vi "TRANCON-Client.vi"() -> ()   [LabVIEW 2020]
uses:
  controls/Rename.ctl
  controls/Load.ctl
  controls/CleanSD.ctl
  controls/Save.ctl
  controls/Del.ctl
  controls/Add.ctl
  controls/Average.ctl
  controls/mylistbox.ctl
  dependecies/XControls/StartButton/StartButton.xctl
  controls/SliderSDII.ctl
  controls/Gauge_pump/Gauge_pump.xctl
  controls/DigitalIndicatorELYSEpulses.ctl
  dependecies/XControls/CellsDL/ControlDL.xctl
  controls/Calc.ctl
  controls/Camera.ctl
  controls/table.ctl
  controls/oscilloscope.ctl
  controls/AllOffOn.ctl
  controls/Fix.ctl
  controls/Scale_up.ctl
  controls/Norm.ctl
  controls/LeftArrow.ctl
  controls/RightArrow.ctl
  controls/Visibility.ctl
  Classes/Control/Control-Client/Control-Client.lvclass
  dependecies/ControlsVIs/Clusters-def/Delays-refs_CLIENT.ctl
  dependecies/ControlsVIs/Clusters-def/graphs_TR.ctl
  dependecies/ControlsVIs/Clusters-def/Graphs_ref_Client.ctl
  dependecies/ControlsVIs/Clusters-def/Controls-with-permissions_CLIENT.ctl
  <vilib>/addons/zeromq/socket_type.ctl
  <vilib>/addons/zeromq/socket_options.ctl
  dependecies/ControlsVIs/Clusters-def/SERVER-Commands.ctl
  dependecies/ControlsVIs/Clusters-def/Message types.ctl
  Classes/Control/Control-Client/Control-Client.lvclass/Control-Client.ctl
  Classes/Experiments/Experiments_group.lvclass/Experiments_group.ctl
  dependecies/ControlsVIs/Clusters-def/Types_of_Graphs-Client.ctl
  Classes/Experiments/Experiment.lvclass/Experiment.ctl
  dependecies/ControlsVIs/Clusters-def/Parameters_measurement_def.ctl
  Classes/Control/Control-Client/methods/Read Group #.vi
  dependecies/globalVarII.vi
  dependecies/globalVarSD.vi
  Classes/Control/Control-Client/Erase color.vi
  Classes/Experiments/Experiments_group.lvclass
  Classes/Control/Control-Server/Control-Server.lvclass
  Classes/Experiments/Experiment.lvclass
  <vilib>/addons/zeromq/zmq_context.lvclass
  <vilib>/addons/zeromq/zmq_socket.lvclass
  <vilib>/addons/zeromq/zeromq.lvlib
panel:
  in  "EXP":bool=TRUE caption="EXP V0/VD2"
  in  "BG type":enum32{"Aver", "Savitzky-Golay"}(radio)=enum."Savitzky-Golay"
  out "BG":cluster{i32[], "Filtered X":dbl[]}[](graph)
  in  "polynom order":i32=10
  in  "side p":i32=10
  in  "aver":bool
  in  "Cut":bool
  in  "right exp":bool
  in  "left exp":bool=TRUE
  in  "Fix":bool
  in  "Up":bool
  in  "Left":bool
  in  "Right":bool
  in  "Numeric":i32=5 min=1 max=50
  in  "scale":dbl=1.01
  in  "timedelays_var":dbl[](array[numeric])=[370.0, 400.0, 450.0, 500.0, 550.0, 600.0, 640.0, 700.0]
  in  "waves_var":dbl[](array[numeric])=[370.0, 400.0, 450.0, 500.0, 550.0, 600.0, 640.0, 700.0]
  in  "Merge":bool
  in  "VD2_calc_abs":bool
  in  "Right shift kinetics":T1
  in  "Left shift kinetics":T2
  in  "Norm Kinetics":T3
  in  "Scale_up":dbl=1.01 format="%#_3f"
  in  "ScaleUp":T4
  in  "Value":dbl=10.0 format="%#_13g"
  in  "ChangeAll":T5
  in  "NaN Correct":T6
  in  "CalcStability":T7
  out "stability":T8(graph)
  in  "X-scale":bool
  out "bytes received":i64 caption="DATA received"
  in  "Group title":string
  in  "Del group exp":T9
  in  "Add group":T10
  out "error out":errorcluster
  in  "Exp name":string
  in  "Clean mode":u16(ring)=1 items=["delete", "approx"]
  in  "Clean":T6
  in  "sigma":dbl=1.4 min=0.0 step=0.1
  in  "BG slider":T11={0.0, 16.0} scale=0.0..15.0
  in  "BG correct":T6
  in  "Add Exp":T10
  in  "Del exp":T9
  in  "Load Exp":T12
  in  "Save exp":T13
  in  "Save":enum32{"Automatic", "User-def"}(ring)
  in  "Rename exp":T14
  in  "Average exp":T15
  in  "times slider":T11={120.7741935483871, 734.8387096774194} scale=0.0..1.0 scale format="%#.1f"
  in  "del spec":i32=2 min=2 step=1
  in  "Del spectrum":T9
  in  "Add spectrum":T10
  out "Spectra":cluster{"Y":dbl[], "Y":dbl[]}[](graph)
  in  "waves slider":T11={434.19354838709677, 734.8387096774194} scale=0.0..1.0 scale format="%#.1f"
  in  "del kin":i32=2 min=2 step=1
  in  "LogY":bool
  in  "Del kinetics":T9
  in  "Add kinetics":T10
  out "Kinetics":cluster{"Y":dbl[], "Y":dbl[]}[](graph)
  in  "Camer connect":bool
  in  "Pump connect":bool
  in  "OSc:Connect":bool
  in  "folder of the day":string="no title"
  out "Power":bool
  in  "DAQmx:Connect":bool
  in  "Unlock":bool
  in  "SERVER:AllConnect":bool caption="All connect"
  in  "DET:Connect":bool
  in  "DL:Connect":bool
  in  "StartButton":bool(xcontrol)
  in  "Server ON/OFF":bool
  in  "selected wavelengths":dbl[](array[numeric])=[370.0, 400.0, 450.0, 500.0, 550.0, 600.0, 640.0, 700.0]
  out "Exp data graph":dbl[][](graph)
  in  "Commentaires exp":string="...Write experiment description..."
  in  "Experiments":T16=[4]
  in  "Group":u16(ring)
  in  "type of probe":enum32{"SC", "OPA"}(radio)
  in  "Tab Control":enum32{"Exp data", "Raw data"}(tab)
  out "TR OD":cluster{dbl[], dbl[]}[](graph)
  in  "CalcAbs":T7
  in  "SaveSC":T13
  in  "RT":bool
  out "TR SC":cluster{dbl[], dbl[]}[](graph)
  in  "correct raw BG":bool
  out "Raw data":cluster{dbl[], dbl[]}[](graph)
  in  "raw bg":i32[](array[numeric])
  out "Raw data BG":cluster{dbl[], dbl[]}[](graph)
  out "Pump":T17(xcontrol)
  in  "visibility":T18
  in  "#cycles_measurement":i32=5 caption="#Cyc" min=1 max=15 step=1
  in  "Define Names":bool
  in  "Repump":bool
  in  "Lockrepump_levels":T19
  out "ELYSE pulses":T20
  in  "channelsOsc":i16[](array[numeric])=[1] min=0 max=3 step=1
  in  "oscilloscopeRead":T21
  out "Oscilloscope":waveform(dbl)[](graph)
  in  "image":T22
  out "Camera":dbl[][](graph)
  out "Total length, ps":dbl=3989.9999999999995 caption="Total"
  out "Kinetics length, ps":dbl=3789.9999999999995 caption="Kinetics" min=-200.0 max=8350.0
  in  "Real zero, ps":dbl=465.0 caption="Real zero"
  in  "remake":bool
  in  "# points":i32=100 min=1 step=1
  in  "OZ, ps":dbl=-250.0
  in  "Step, ps":dbl=15.0 min=-100.0 max=5000.0 step=1.0
  in  "TableLoad":T23
  out "Delays Graph":cluster{i32[], "array w/ subset deleted":dbl[]}(graph)
  in  "DAQmx:FaradayCup":bool caption="Accelerator shutter"
  out "Alarm":bool
  in  "DAQmx:RelayKeyHeater":bool caption="Accelerator shutter"
  in  "DAQmx:AcceleratorShutter":bool caption="Accelerator shutter"
  in  "DAQmx:LaserShutter":bool
  in  "Time, ms":dbl=10.0 min=1.0 max=150.0
  in  "DAQmx:MoveCrystal":bool
  in  "Start measurement":bool
  in  "Wavelength fix":dbl=640.0 caption="wave fix"
  in  "ODmax":dbl=0.5
  in  "ODmin":dbl=-0.5
  in  "# par point":i32=10 caption="# PP" min=1 max=100 step=1
  out "# current":i32 caption="#"
  out "RDT, ps":dbl=3789.9999999999995 caption="RDT"
  in  "Aq contol":enum32{"fixed", "automatic", "fixed-auto"}(radio)
  in  "ControlDL":cluster{"positions":dbl[]}(xcontrol)
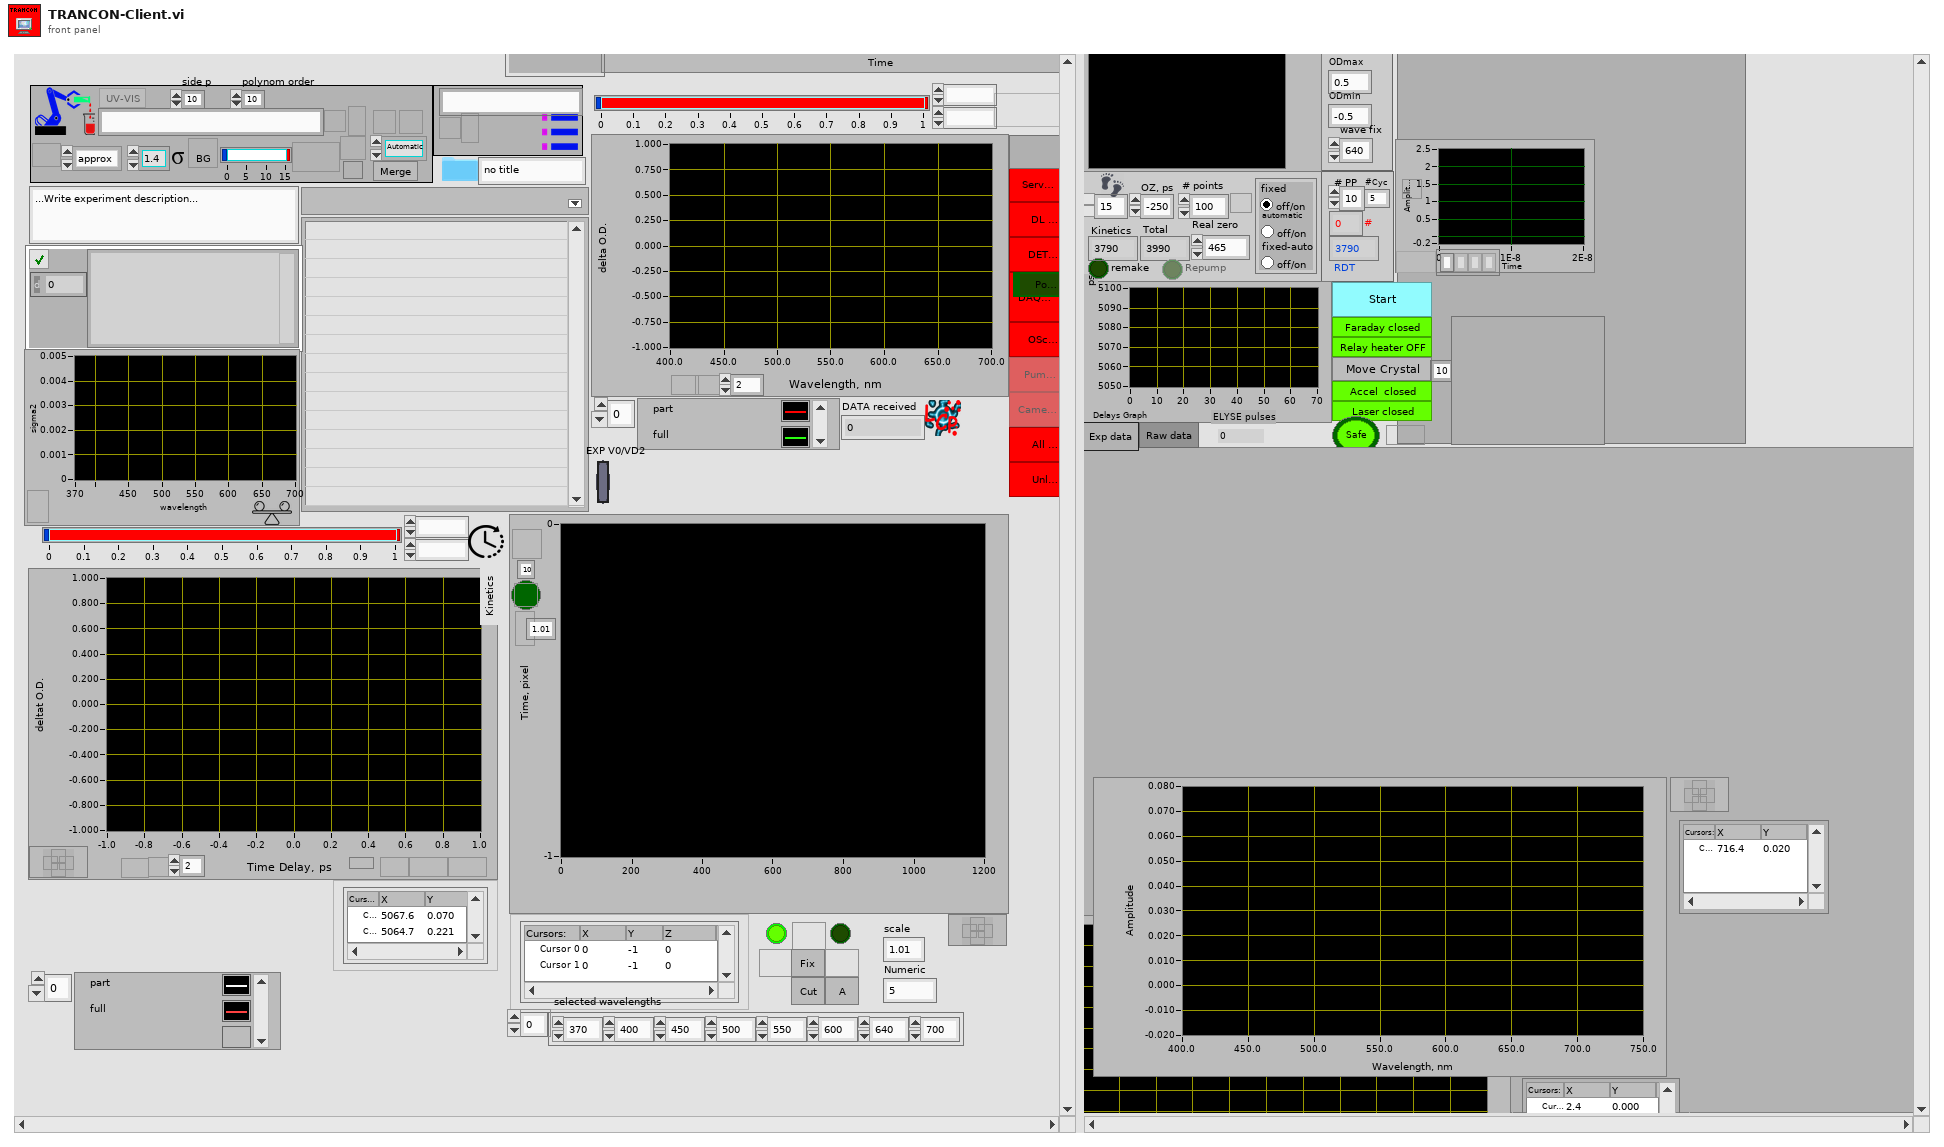
[diagram p1: front panel]
types:
  T1 = typedef "RightArrow.ctl" = bool
  T2 = typedef "LeftArrow.ctl" = bool
  T3 = typedef "Norm.ctl" = bool
  T4 = typedef "Scale_up.ctl" = bool
  T5 = typedef "AllOffOn.ctl" = bool
  T6 = typedef "CleanSD.ctl" = bool
  T7 = typedef "Calc.ctl" = bool
  T8 = cluster{"wavelengths":dbl[], "wavelengths":dbl[]}[]
  T9 = typedef "Del.ctl" = bool
  T10 = typedef "Add.ctl" = bool
  T11 = typedef "SliderSDII.ctl" = cluster{dbl, dbl}
  T12 = typedef "Load.ctl" = bool
  T13 = typedef "Save.ctl" = bool
  T14 = typedef "Rename.ctl" = bool
  T15 = typedef "Average.ctl" = bool
  T16 = typedef "mylistbox.ctl" = i32[]
  T17 = cluster{"Data":dbl, "direction":bool, "start/stop":bool}
  T18 = typedef "Visibility.ctl" = bool
  T19 = typedef "Fix.ctl" = bool
  T20 = typedef "DigitalIndicatorELYSEpulses.ctl" = i64
  T21 = typedef "oscilloscope.ctl" = bool
  T22 = typedef "Camera.ctl" = bool
  T23 = typedef "table.ctl" = bool
  T24 = cluster{"waves slider":refnum<vi>, "times slider":refnum<vi>}
  T25 = typedef "Control-Client.lvclass/Controls-with-permissions_CLIENT.ctl" = cluster{"Server ON/OFF":refnum<vi>, "Detector connect":refnum<vi>, "DL connect":refnum<vi>, "DAQmx connect":refnum<vi>, "All connect":refnum<vi>, "Start measurement":refnum<vi>, "Move Crystal":refnum<vi>, "Relay key heater":refnum<vi>, "Laser Shutter":refnum<vi>, "Accelerator Shutter":refnum<vi>, "Power":refnum<vi>, "Unlock":refnum<vi>, "RT":refnum<vi>, "Faraday Cup":refnum<vi>, "Osc connect":refnum<vi>, "ELYSE pulses":refnum<vi>, "Cells":refnum<vi>, "Pump":refnum<vi>, "# par point":refnum<vi>, "Alarm":refnum<vi>, "oscilloscopeRead":refnum<vi>, "WCM_state":refnum<vi>, "ControlDL":refnum<vi>}
  T26 = typedef "Control-Client.lvclass/Graphs_ref_Client.ctl" = cluster{"Exp data graph ref":refnum<vi>, "Kinetics graph ref":refnum<vi>, "Spectrum graph ref":refnum<vi>, "cluster graph TR":T27, "Delays Graph":refnum<vi>, "Oscilloscope":refnum<vi>}
  T27 = typedef "graphs_TR.ctl" = cluster{"TR SC":refnum<vi>, "TR OD":refnum<vi>, "Raw data":refnum<vi>, "Raw data BG":refnum<vi>}
  T28 = typedef "Control-Client.lvclass/Delays-refs_CLIENT.ctl" = cluster{"# points":refnum<vi>, "Step, ps":refnum<vi>, "OZ, ps":refnum<vi>, "# current":refnum<vi>, "RDT, ps":refnum<vi>, "Total length, ps":refnum<vi>, "Kinetics length, ps":refnum<vi>, "Real zero, ps":refnum<vi>, "# par point":refnum<vi>}
  T29 = cluster{"error out":refnum<vi>, "Experiments":refnum<vi>, "Group":refnum<vi>, "Commentaires exp":refnum<vi>}
  T30 = typedef "zeromq.lvlib/socket_options.ctl" = enum8{"NONE", "ZMQ_HWM", "<2>", "ZMQ_SWAP", "ZMQ_AFFINITY", "ZMQ_ROUTING_ID", "ZMQ_SUBSCRIBE", "ZMQ_UNSUBSCRIBE", "ZMQ_RATE", "ZMQ_RECOVERY_IVL", "ZMQ_MCAST_LOOP", "ZMQ_SNDBUF", "ZMQ_RCVBUF", "ZMQ_RCVMORE", "ZMQ_FD", "ZMQ_EVENTS", "ZMQ_TYPE", "ZMQ_LINGER", "ZMQ_RECONNECT_IVL", "ZMQ_BACKLOG", "ZMQ_RECOVERY_IVL_MSEC", "ZMQ_RECONNECT_IVL_MAX", "ZMQ_MAXMSGSIZE", "ZMQ_SNDHWM", "ZMQ_RCVHWM", "ZMQ_MULTICAST_HOPS", "<26>", "ZMQ_RCVTIMEO", "ZMQ_SNDTIMEO", "<29>", "<30>", "ZMQ_IPV4ONLY", "ZMQ_LAST_ENDPOINT", "ZMQ_ROUTER_MANDATORY", "ZMQ_TCP_KEEPALIVE", "ZMQ_TCP_KEEPALIVE_CNT", "ZMQ_TCP_KEEPALIVE_IDLE", "ZMQ_TCP_KEEPALIVE_INTVL", "ZMQ_TCP_ACCEPT_FILTER", "ZMQ_IMMEDIATE", "ZMQ_XPUB_VERBOSE", "ZMQ_ROUTER_RAW", "ZMQ_IPV6", "ZMQ_MECHANISM", "ZMQ_PLAIN_SERVER", "ZMQ_PLAIN_USERNAME", "ZMQ_PLAIN_PASSWORD", "ZMQ_CURVE_SERVER", "ZMQ_CURVE_PUBLICKEY", "ZMQ_CURVE_SECRETKEY", "ZMQ_CURVE_SERVERKEY", "ZMQ_PROBE_ROUTER", "ZMQ_REQ_CORRELATE", "ZMQ_REQ_RELAXED", "ZMQ_CONFLATE", "ZMQ_ZAP_DOMAIN", "ZMQ_ROUTER_HANDOVER", "ZMQ_TOS", "ZMQ_IPC_FILTER_PID", "ZMQ_IPC_FILTER_UID", "ZMQ_IPC_FILTER_GID", "ZMQ_CONNECT_ROUTING_ID", "ZMQ_GSSAPI_SERVER", "ZMQ_GSSAPI_PRINCIPAL", "ZMQ_GSSAPI_SERVICE_PRINCIPAL", "ZMQ_GSSAPI_PLAINTEXT", "ZMQ_HANDSHAKE_IVL", "<67>", "ZMQ_SOCKS_PROXY", "ZMQ_XPUB_NODROP", "ZMQ_BLOCKY", "ZMQ_XPUB_MANUAL", "ZMQ_XPUB_WELCOME_MSG", "ZMQ_STREAM_NOTIFY", "ZMQ_INVERT_MATCHING", "ZMQ_HEARTBEAT_IVL", "ZMQ_HEARTBEAT_TTL", "ZMQ_HEARTBEAT_TIMEOUT", "ZMQ_XPUB_VERBOSER", "ZMQ_CONNECT_TIMEOUT", "ZMQ_TCP_MAXRT", "ZMQ_THREAD_SAFE", "<82>", "<83>", "ZMQ_MULTICAST_MAXTPDU", "ZMQ_VMCI_BUFFER_SIZE", "ZMQ_VMCI_BUFFER_MIN_SIZE", "ZMQ_VMCI_BUFFER_MAX_SIZE", "ZMQ_VMCI_CONNECT_TIMEOUT", "ZMQ_USE_FD", "ZMQ_GSSAPI_PRINCIPAL_NAMETYPE", "ZMQ_GSSAPI_SERVICE_PRINCIPAL_NAMETYPE", "ZMQ_BINDTODEVICE", "ZMQ_ZAP_ENFORCE_DOMAIN", "ZMQ_LOOPBACK_FASTPATH", "ZMQ_METADATA", "ZMQ_MULTICAST_LOOP", "ZMQ_ROUTER_NOTIFY"}
  T31 = typedef "zeromq.lvlib/socket_type.ctl" = enum8{"ZMQ_PAIR", "ZMQ_PUB", "ZMQ_SUB", "ZMQ_REQ", "ZMQ_REP", "ZMQ_DEALER", "ZMQ_ROUTER", "ZMQ_PULL", "ZMQ_PUSH", "ZMQ_XPUB", "ZMQ_XSUB", "ZMQ_STREAM", "ZMQ_SERVER", "ZMQ_CLIENT", "ZMQ_RADIO", "ZMQ_DISH", "ZMQ_GATHER", "ZMQ_SCATTER", "ZMQ_DGRAM"}
  T32 = typedef "Message types.ctl" = string
  T33 = typedef "Control-Server.lvclass/SERVER-Commands.ctl" = string
  T34 = cluster{"Fix":bool, "DeltaT":dbl, "#points":i32, "Delay":dbl, "output cluster":cluster{"From Time":dbl, "To Time":dbl, "From Wave":dbl, "To Wave":dbl}}
  T35 = typedef "Control-Client.lvclass/Types_of_Graphs-Client.ctl" = string
  T36 = typedef "Parameters_measurement_def.ctl" = cluster{"ODmin":dbl, "ODmax":dbl, "Aq contol":enum32{"fixed", "automatic", "fixed-auto"}, "Wavelength_fix_index":i32, "repump_limits":cluster{"repump_min":dbl, "repump_max":dbl, "repump_value":dbl}, "repump_correction":bool, "#cycles max":i32}
  T37 = enum32{"Invalid", "Standard", "Closed", "Hidden", "Minimized", "Maximized"}
  T38 = cluster{"Value":string, "Value":string, cluster{dbl, dbl, dbl, dbl}}
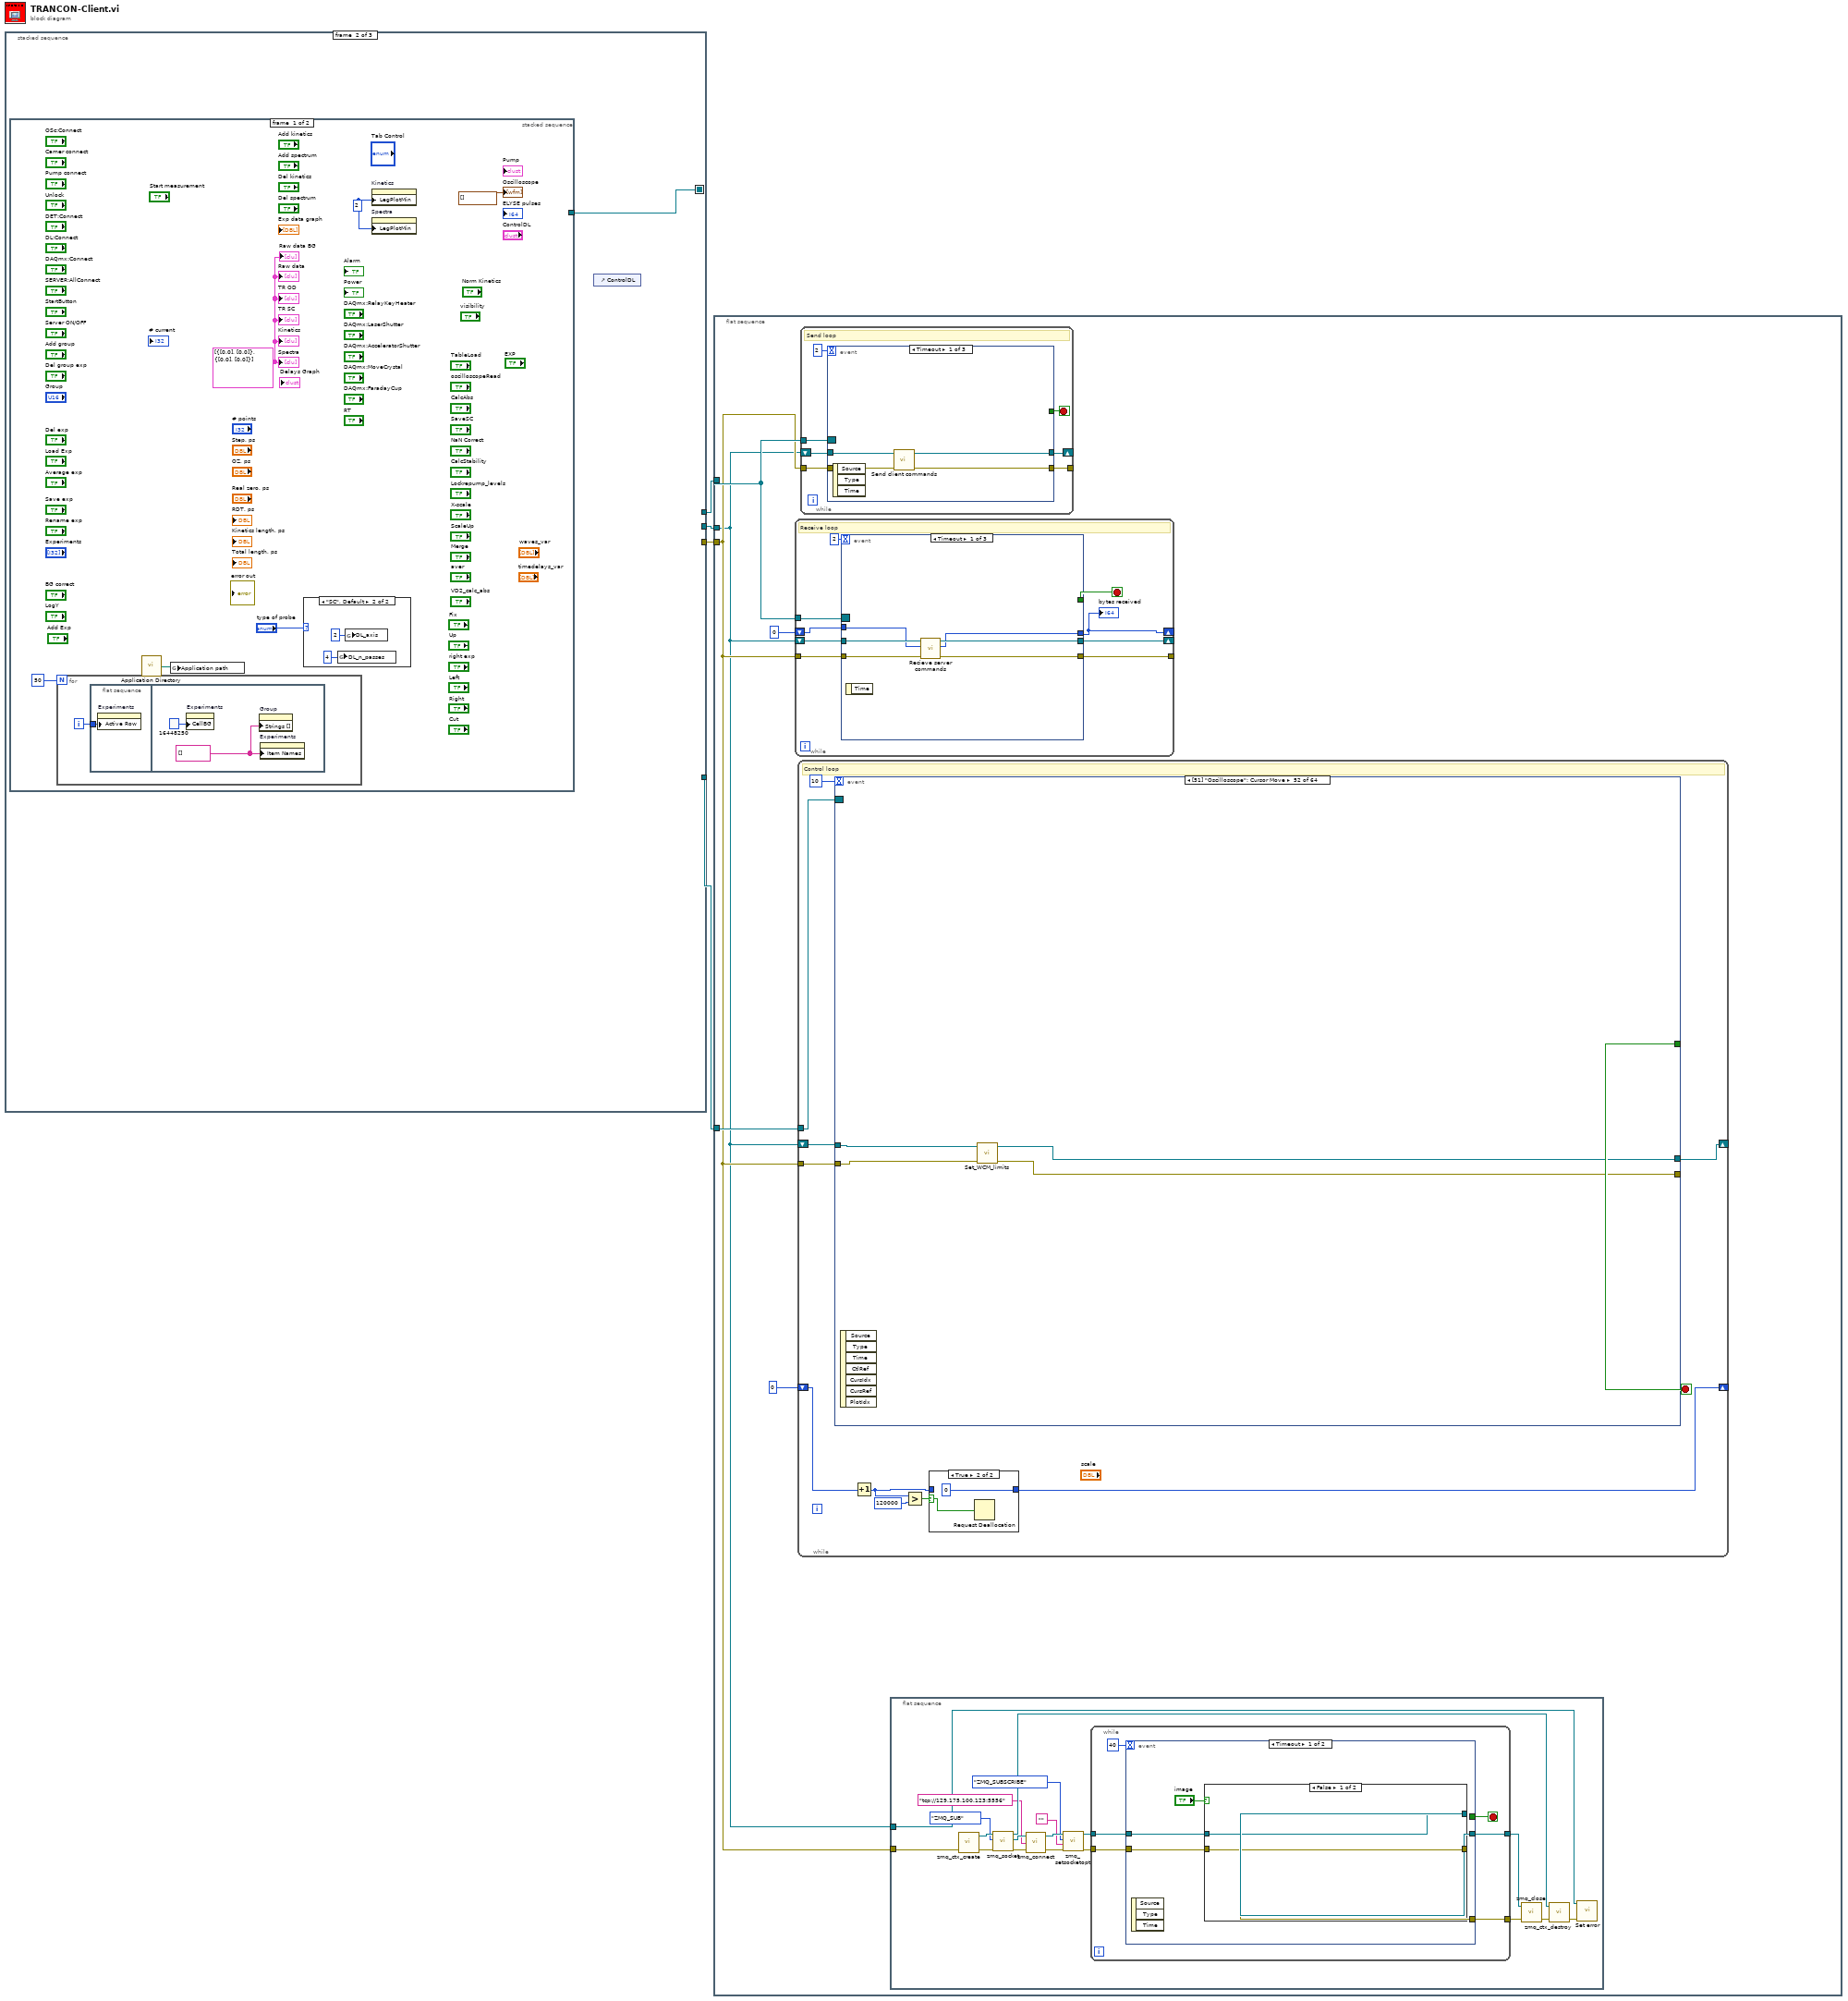
[diagram p0: block diagram]
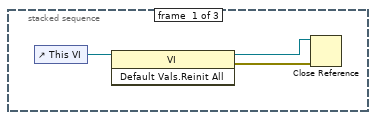
[diagram p2: hidden frame]
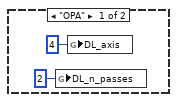
[diagram p3: hidden frame]
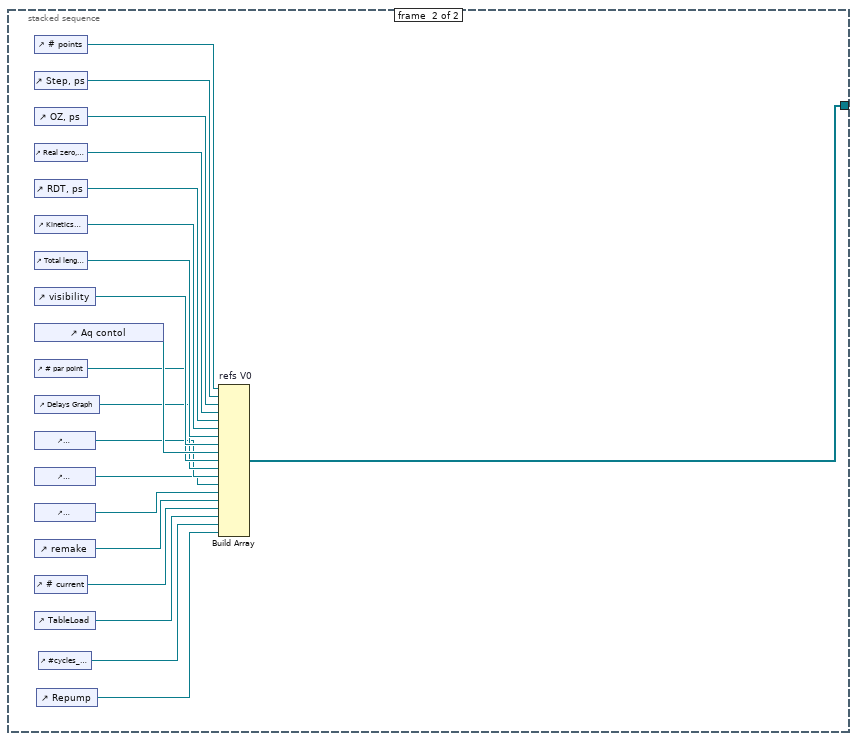
[diagram p4: hidden frame]
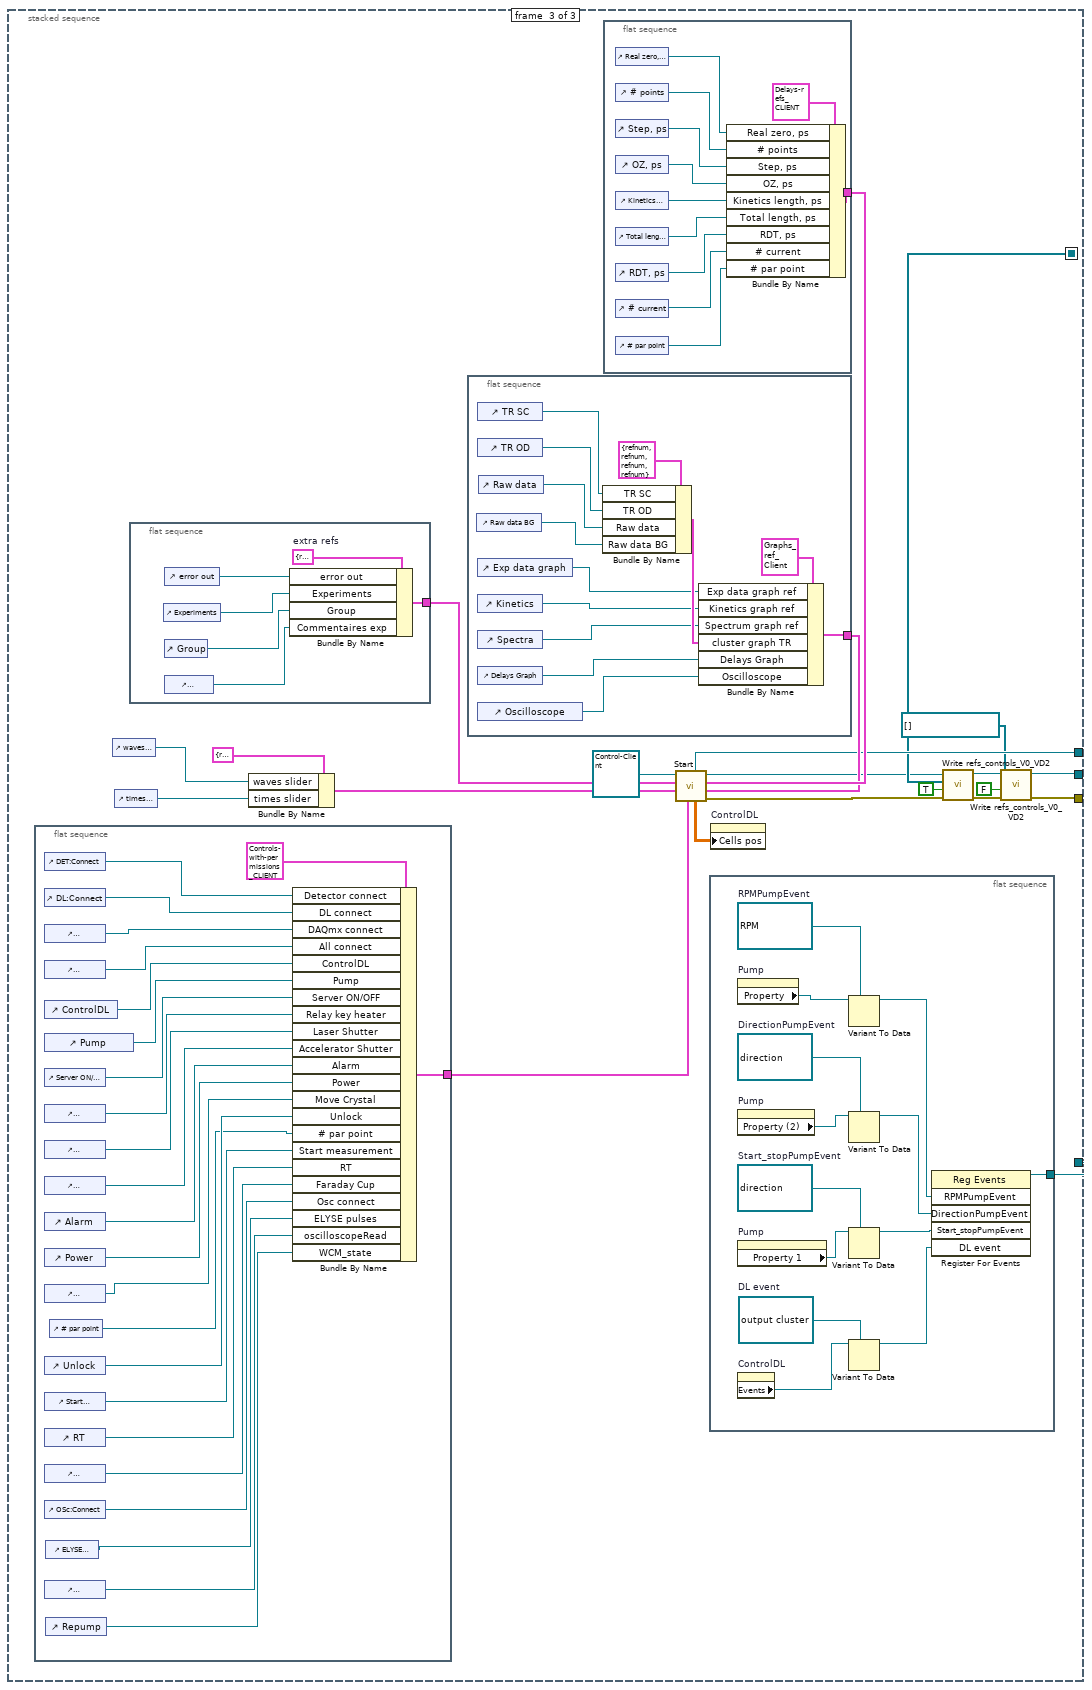
[diagram p5: hidden frame]
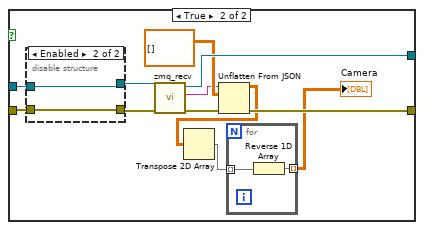
[diagram p6: hidden frame]
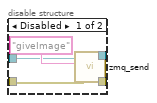
[diagram p7: hidden frame]
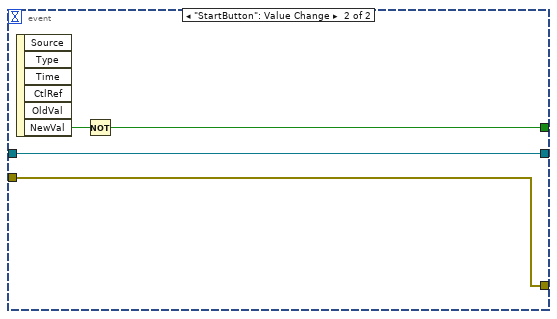
[diagram p8: hidden frame]
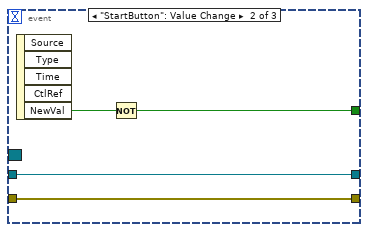
[diagram p9: hidden frame]
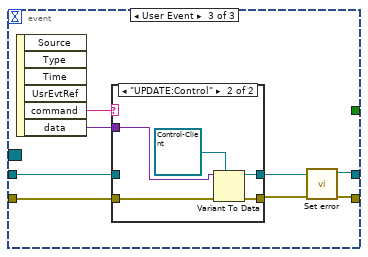
[diagram p10: hidden frame]
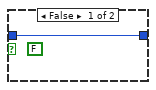
[diagram p12: hidden frame]
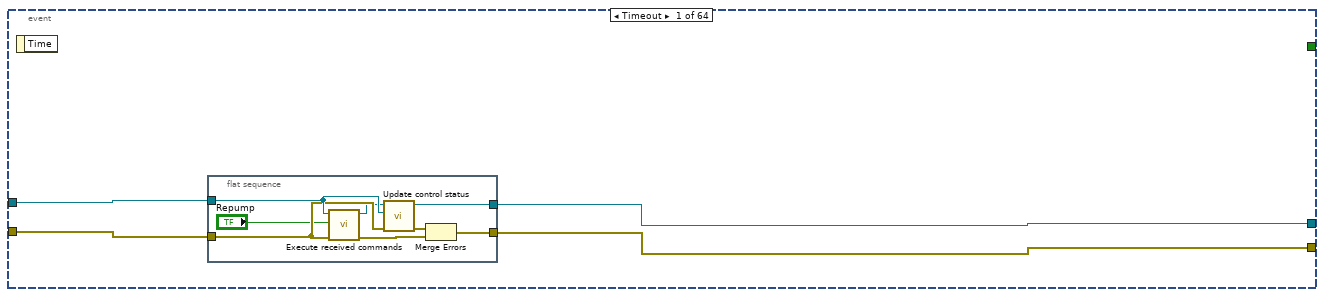
[diagram p13: hidden frame]
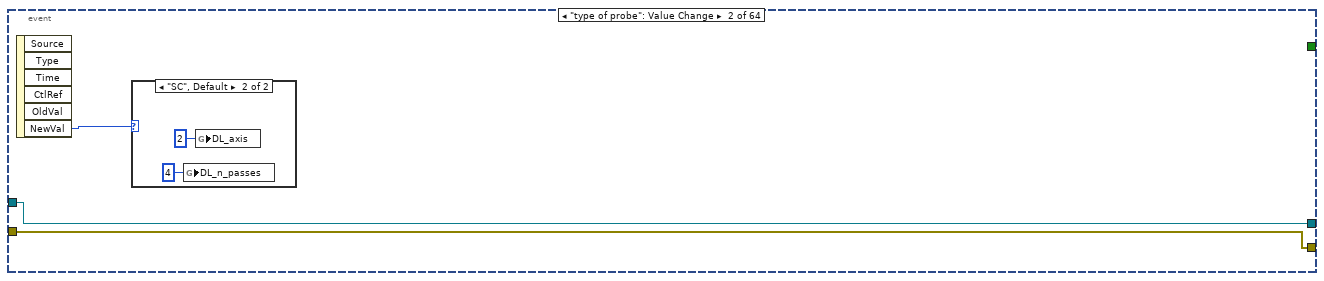
[diagram p14: hidden frame]
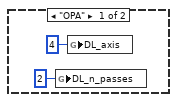
[diagram p15: hidden frame]
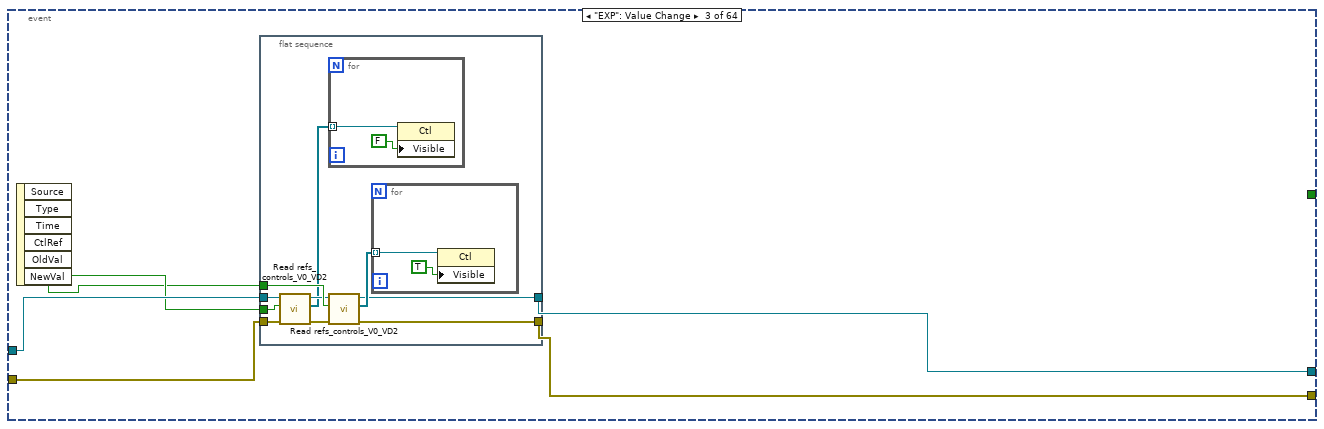
[diagram p16: hidden frame]
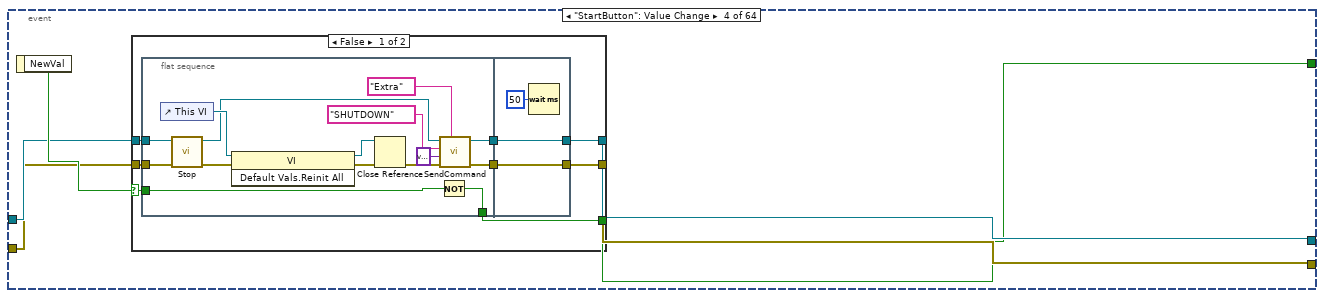
[diagram p17: hidden frame]
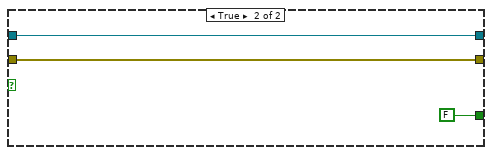
[diagram p18: hidden frame]
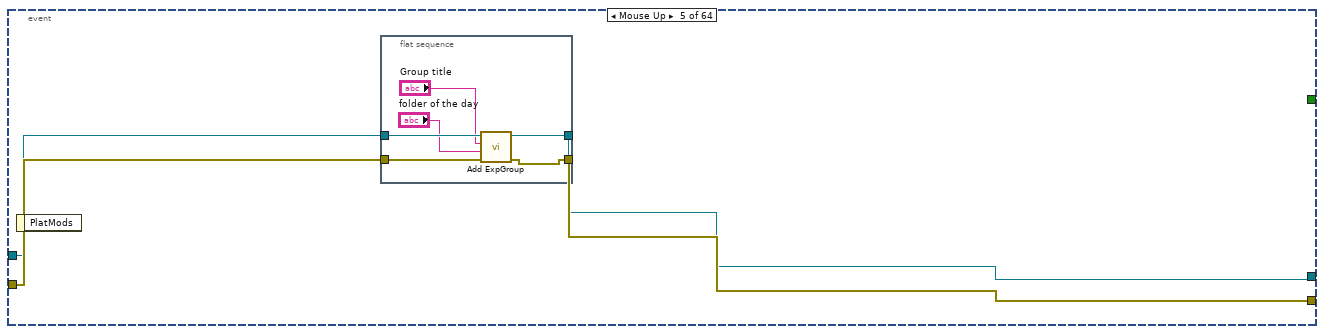
[diagram p19: hidden frame]
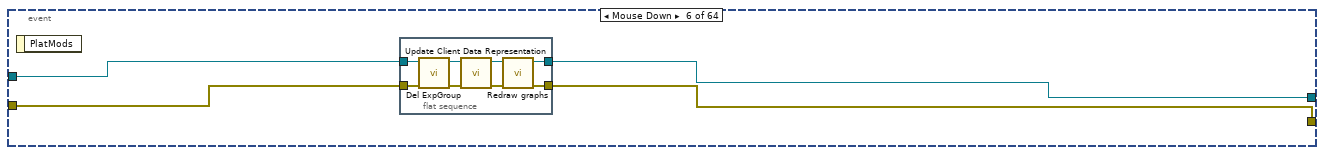
[diagram p20: hidden frame]
diagram:
  n1 = stacked-sequence {
    seq-local: [_ w8 _] -> [_ _ w51]
    tunnel: [_ _ w47] -> w4
    tunnel: [_ _ w46] -> w1
    tunnel: [_ _ w54] -> w3
    tunnel: [_ _ w62] -> w2
    frame #0 {
      n2 = control-ref of="This VI"() -> (w7:refnum<vi>)
      n3 = invoke class="VI" method="Default Vals.Reinit All"(reference=w7) -> (reference out=w6:refnum<vi>, error out=w5:errorcluster)  [unwired: 2 in, 1 out]
      n4 = Close Reference(reference=w6, error in (no error)=w5) -> ()  [unwired: 1 out]
    }
    frame #1 {
      n5 = stacked-sequence {
        tunnel: [_ w32] -> w8
        frame #0 {
          w10 = cluster{dbl[], dbl[]}[] [{[0.0], [0.0]}, {[0.0], [0.0]}] ("Kinetics")
          w12 = u32 2 ("Legend:Plot Minimum")
          n6 = for {
            N: 50 -> [_]
            i -> [w19]
            n7 = flat-sequence {
              tunnel: w19 -> [w20]
              frame #0 {
                n8 = property on="Experiments" class="LstBox (strict)"("Active Row"=w20) -> ()  [unwired: 2 in, 2 out]
              }
              frame #1 {
                w21 = string[] [] ("Item Names")
                n9 = property on="Experiments" class="LstBox (strict)"("CellBG"=u32 16448250) -> ()  [unwired: 2 in, 2 out]
                n10 = property on="Group" class="Ring (strict)"("Strings []"=w21) -> ()  [unwired: 2 in, 2 out]
                n11 = property on="Experiments" class="LstBox (strict)"("Item Names"=w21) -> ()  [unwired: 2 in, 2 out]
              }
            }
          }
          n12 = call <vilib>:"Application Directory.vi"() -> ("Application Directory"=w14:path)
          n13 = global write "globalVarSD.vi" "Application path"(w14) -> ()
          n14 = case shown="\"SC\", Default" "type of probe" {
            frame "OPA" {
              n15 = global write "globalVarII.vi" "DL_n_passes"(2 ("DL_n_passes")) -> ()
              n16 = global write "globalVarII.vi" "DL_axis"(4 ("DL_axis")) -> ()
            }
            frame "SC", Default {
              n17 = global write "globalVarII.vi" "DL_n_passes"(4 ("DL_n_passes")) -> ()
              n18 = global write "globalVarII.vi" "DL_axis"(2 ("DL_axis")) -> ()
            }
          }
          n19 = property on="Kinetics" class="XYGraph (strict)"("LegPlotMin"=w12) -> ()  [unwired: 2 in, 2 out]
          n20 = property on="Spectra" class="XYGraph (strict)"("LegPlotMin"=w12) -> ()  [unwired: 2 in, 2 out]
          "TR OD" <- w10
          "TR SC" <- w10
          "Spectra" <- w10
          "Kinetics" <- w10
          "Oscilloscope" <- waveform(dbl)[] [] ("Data")
          "Raw data" <- w10
          "Raw data BG" <- w10
        }
        frame #1 {
          n21 = control-ref of="# points"() -> (w42:refnum<vi>)
          n22 = control-ref of="Step, ps"() -> (w41:refnum<vi>)
          n23 = control-ref of="OZ, ps"() -> (w40:refnum<vi>)
          n24 = control-ref of="Real zero, ps"() -> (w39:refnum<vi>)
          n25 = control-ref of="RDT, ps"() -> (w38:refnum<vi>)
          n26 = control-ref of="Kinetics length, ps"() -> (w37:refnum<vi>)
          n27 = control-ref of="Total length, ps"() -> (w36:refnum<vi>)
          n28 = control-ref of="visibility"() -> (w35:refnum<vi>)
          n29 = control-ref of="Aq contol"() -> (w34:refnum<vi>)
          n30 = control-ref of="# par point"() -> (w33:refnum<vi>)
          n31 = control-ref of="Delays Graph"() -> (w31:refnum<vi>)
          n32 = control-ref of="DAQmx:MoveCrystal"() -> (w30:refnum<vi>)
          n33 = control-ref of="DAQmx:AcceleratorShutter"() -> (w29:refnum<vi>)
          n34 = control-ref of="DAQmx:LaserShutter"() -> (w28:refnum<vi>)
          n35 = control-ref of="remake"() -> (w27:refnum<vi>)
          n36 = control-ref of="# current"() -> (w26:refnum<vi>)
          n37 = control-ref of="TableLoad"() -> (w25:refnum<vi>)
          n38 = control-ref of="Repump"() -> (w23:refnum<vi>)
          n39 = control-ref of="#cycles_measurement"() -> (w24:refnum<vi>)
          n40 = Build Array "refs V0"(w42, w41, w40, w39, w38, w37, w36, w35, w34, w33, w31, w30, w29, w28, w27, w26, w25, w24, w23) -> (w32:refnum<vi>[])
        }
      }
      n41 = control-ref of="ControlDL"() -> ()  [unwired: 1 out]
    }
    frame #2 {
      n42 = flat-sequence {
        tunnel: [w71] -> w57
        frame #0 {
          n43 = control-ref of="DET:Connect"() -> (w94:refnum<vi>)
          n44 = control-ref of="DL:Connect"() -> (w93:refnum<vi>)
          n45 = control-ref of="DAQmx:Connect"() -> (w92:refnum<vi>)
          n46 = control-ref of="SERVER:AllConnect"() -> (w91:refnum<vi>)
          n47 = control-ref of="ControlDL"() -> (w78:refnum<vi>)
          n48 = control-ref of="Pump"() -> (w77:refnum<vi>)
          n49 = control-ref of="Server ON/OFF"() -> (w90:refnum<vi>)
          n50 = control-ref of="DAQmx:RelayKeyHeater"() -> (w89:refnum<vi>)
          n51 = control-ref of="DAQmx:LaserShutter"() -> (w88:refnum<vi>)
          n52 = control-ref of="DAQmx:AcceleratorShutter"() -> (w87:refnum<vi>)
          n53 = control-ref of="Alarm"() -> (w75:refnum<vi>)
          n54 = control-ref of="Power"() -> (w86:refnum<vi>)
          n55 = control-ref of="DAQmx:MoveCrystal"() -> (w85:refnum<vi>)
          n56 = control-ref of="Unlock"() -> (w83:refnum<vi>)
          n57 = control-ref of="Start measurement"() -> (w82:refnum<vi>)
          n58 = control-ref of="RT"() -> (w81:refnum<vi>)
          n59 = control-ref of="DAQmx:FaradayCup"() -> (w80:refnum<vi>)
          n60 = control-ref of="OSc:Connect"() -> (w79:refnum<vi>)
          n61 = control-ref of="oscilloscopeRead"() -> (w74:refnum<vi>)
          n62 = control-ref of="ELYSE pulses"() -> (w73:refnum<vi>)
          n63 = control-ref of="Repump"() -> (w72:refnum<vi>)
          n64 = control-ref of="# par point"() -> (w76:refnum<vi>)
          n65 = Bundle By Name(cluster=T25 {"Server ON/OFF"=refnum, "Detector connect"=refnum, "DL connect"=refnum, "DAQmx connect"=refnum, "All connect"=refnum, "Start measurement"=refnum, "Move Crystal"=refnum, "Relay key heater"=refnum, "Laser Shutter"=refnum, "Accelerator Shutter"=refnum, "Power"=refnum, "Unlock"=refnum, "RT"=refnum, "Faraday Cup"=refnum, "Osc connect"=refnum, "ELYSE pulses"=refnum, "Cells"=refnum, "Pump"=refnum, "# par point"=refnum, "Alarm"=refnum, "oscilloscopeRead"=refnum, "WCM_state"=refnum, "ControlDL"=refnum} ("output cluster"), "Detector connect"=w94, "DL connect"=w93, "DAQmx connect"=w92, "All connect"=w91, "ControlDL"=w78, "Pump"=w77, "Server ON/OFF"=w90, "Relay key heater"=w89, "Laser Shutter"=w88, "Accelerator Shutter"=w87, "Alarm"=w75, "Power"=w86, "Move Crystal"=w85, "Unlock"=w83, "# par point"=w76, "Start measurement"=w82, "RT"=w81, "Faraday Cup"=w80, "Osc connect"=w79, "ELYSE pulses"=w73, "oscilloscopeRead"=w74, "WCM_state"=w72) -> (w71:T25)
        }
      }
      n66 = control-ref of="waves slider"() -> (w60:refnum<vi>)
      n67 = control-ref of="times slider"() -> (w61:refnum<vi>)
      n68 = flat-sequence {
        tunnel: [w65] -> w55
        frame #0 {
          w70 = T29 {"error out"=refnum, "Experiments"=refnum, "Group"=refnum, "Commentaires exp"=refnum}  # extra refs
          n69 = control-ref of="Experiments"() -> (w68:refnum<vi>)
          n70 = control-ref of="error out"() -> (w69:refnum<vi>)
          n71 = control-ref of="Group"() -> (w67:refnum<vi>)
          n72 = control-ref of="Commentaires exp"() -> (w66:refnum<vi>)
          n73 = Bundle By Name(cluster=w70, "error out"=w69, "Experiments"=w68, "Group"=w67, "Commentaires exp"=w66) -> (w65:T29)
        }
      }
      n74 = Bundle By Name(cluster=T24 {"waves slider"=refnum, "times slider"=refnum}, "waves slider"=w60, "times slider"=w61) -> (w59:T24)
      n75 = flat-sequence {
        tunnel: [w103] -> w56
        frame #0 {
          n76 = control-ref of="Raw data BG"() -> (w95:refnum<vi>)
          n77 = control-ref of="TR SC"() -> (w106:refnum<vi>)
          n78 = control-ref of="TR OD"() -> (w105:refnum<vi>)
          n79 = control-ref of="Exp data graph"() -> (w98:refnum<vi>)
          n80 = control-ref of="Kinetics"() -> (w100:refnum<vi>)
          n81 = control-ref of="Spectra"() -> (w99:refnum<vi>)
          n82 = control-ref of="Delays Graph"() -> (w101:refnum<vi>)
          n83 = control-ref of="Oscilloscope"() -> (w97:refnum<vi>)
          n84 = control-ref of="Raw data"() -> (w96:refnum<vi>)
          n85 = Bundle By Name(cluster=T27 {"TR SC"=refnum, "TR OD"=refnum, "Raw data"=refnum, "Raw data BG"=refnum} ("cluster de sortie"), "TR SC"=w106, "TR OD"=w105, "Raw data"=w96, "Raw data BG"=w95) -> (w102:T27)
          n86 = Bundle By Name(cluster=T26 {"Exp data graph ref"=refnum, "Kinetics graph ref"=refnum, "Spectrum graph ref"=refnum, "cluster graph TR"={"TR SC"=refnum, "TR OD"=refnum, "Raw data"=refnum, "Raw data BG"=refnum}, "Delays Graph"=refnum, "Oscilloscope"=refnum} ("Graph refs"), "Exp data graph ref"=w98, "Kinetics graph ref"=w100, "Spectrum graph ref"=w99, "cluster graph TR"=w102, "Delays Graph"=w101, "Oscilloscope"=w97) -> (w103:T26)
        }
      }
      n87 = flat-sequence {
        tunnel: [w109] -> w58
        frame #0 {
          n88 = control-ref of="Real zero, ps"() -> (w113:refnum<vi>)
          n89 = control-ref of="# points"() -> (w114:refnum<vi>)
          n90 = control-ref of="Step, ps"() -> (w115:refnum<vi>)
          n91 = control-ref of="OZ, ps"() -> (w116:refnum<vi>)
          n92 = control-ref of="Kinetics length, ps"() -> (w117:refnum<vi>)
          n93 = control-ref of="Total length, ps"() -> (w118:refnum<vi>)
          n94 = control-ref of="RDT, ps"() -> (w111:refnum<vi>)
          n95 = control-ref of="# current"() -> (w110:refnum<vi>)
          n96 = control-ref of="# par point"() -> (w108:refnum<vi>)
          n97 = Bundle By Name(cluster=T28 {"# points"=refnum, "Step, ps"=refnum, "OZ, ps"=refnum, "# current"=refnum, "RDT, ps"=refnum, "Total length, ps"=refnum, "Kinetics length, ps"=refnum, "Real zero, ps"=refnum, "# par point"=refnum}, "Real zero, ps"=w113, "# points"=w114, "Step, ps"=w115, "OZ, ps"=w116, "Kinetics length, ps"=w117, "Total length, ps"=w118, "RDT, ps"=w111, "# current"=w110, "# par point"=w108) -> (w109:T28)
        }
      }
      n98 = call "Start.vi"("Graph refs"=w56, "Delays refs"=w58, "buttons refs"=w57, "Slider cluster"=w59, "extra refs"=w55, "Control-Client in"=refnum<class "Control-Client.lvclass"> refnum) -> ("error out"=w52:errorcluster, "Control-Client out"=w49:refnum<class "Control-Client.lvclass">, "preset pos"=w53:dbl[][], "ControlEventCom event"=w54:refnum<event-registration>)  [unwired: 2 in]
      n99 = flat-sequence {
        tunnel: [w131] -> w62
        frame #0 {
          w119 = refnum<user-event> refnum  # DL event
          w124 = refnum<user-event> refnum  # Start_stopPumpEvent
          w127 = refnum<user-event> refnum  # DirectionPumpEvent
          w129 = refnum<user-event> refnum  # RPMPumpEvent
          n100 = property on="Pump" class="Gauge_pump (strict)"() -> ("Property"=w130:refnum<user-event>)  [unwired: 2 in, 2 out]
          n101 = property on="Pump" class="Gauge_pump (strict)"() -> ("Property (2)"=w126:refnum<user-event>)  [unwired: 2 in, 2 out]
          n102 = property on="Pump" class="Gauge_pump (strict)"() -> ("Property 1"=w123:refnum<user-event>)  [unwired: 2 in, 2 out]
          n103 = property on="ControlDL" class="ControlDL (strict)"() -> ("Events"=w120:refnum<user-event>)  [unwired: 2 in, 2 out]
          n104 = Variant To Data(type=w129, Variant=w130) -> (data=w128:refnum<user-event>)  [unwired: 1 in, 1 out]
          n105 = Variant To Data(type=w127, Variant=w126) -> (data=w125:refnum<user-event>)  [unwired: 1 in, 1 out]
          n106 = Variant To Data(type=w124, Variant=w123) -> (data=w122:refnum<user-event>)  [unwired: 1 in, 1 out]
          n107 = Variant To Data(type=w119, Variant=w120) -> (data=w121:refnum<user-event>)  [unwired: 1 in, 1 out]
          n108 = register-events(w128, w125, w122, w121) -> (reference out=w131:refnum<event-registration>)  [unwired: 2 in, 1 out]
        }
      }
      n109 = property on="ControlDL" class="ControlDL (strict)"("Cells pos"=w53) -> ()  [unwired: 2 in, 2 out]
      n110 = call-dynamic "Write refs_controls_V0_VD2.vi"("error in (no error)"=w52, "EXP"=TRUE, "refs_controls_V0"=w51, "Control-Client in"=w49) -> ("error out"=w48:errorcluster, "Control-Client out"=w45:refnum<class "Control-Client.lvclass">)  [unwired: 6 in]
      n111 = call-dynamic "Write refs_controls_V0_VD2.vi"("error in (no error)"=w48, "EXP"=FALSE, "refs_controls_V0"=refnum<vi>[] [], "Control-Client in"=w45) -> ("error out"=w47:errorcluster, "Control-Client out"=w46:refnum<class "Control-Client.lvclass">)  [unwired: 6 in]
    }
  }
  n112 = flat-sequence {
    tunnel: w4 -> [w135]
    tunnel: w1 -> [w134]
    tunnel: w3 -> [w137]
    tunnel: w2 -> [w136]
    frame #0 {
      n113 = while {
        shift-right: [w1162] -> _
        shift-left: w134 -> [w1165]
        tunnel: w137 -> [w1161]
        tunnel: w135 -> [w1164]
        tunnel: [w1163] -> _
        shift-right: [w1158] -> _
        shift-left: 0 -> [w1159]
        stop <- w1166 stop-if-true
        # "Receive loop"
        n114 = event shown="[0] Timeout" {
          selector: w1161 -> [_ _ _]
          dyn-events: _ -> [_ _ _]
          timeout: 2 -> [_ _ _]
          tunnel: [_ w1174 _] -> w1166
          tunnel: w1165 -> [w1172 w1177 w1184]
          tunnel: w1164 -> [w1171 w1176 w1183]
          tunnel: [w1169 w1176 w1179] -> w1163
          tunnel: [w1170 w1177 w1180] -> w1162
          tunnel: [w1167 w1173 w1178] -> w1158
          tunnel: w1159 -> [w1168 w1173 w1178]
          event Timeout {
            n115 = event-data() -> ()  [unwired: 1 in, 1 out]
            n116 = call "Recieve server commands.vi"("error in (no error)"=w1171, "bytes in"=w1168, "Control-Client in"=w1172) -> ("error out"=w1169:errorcluster, "bytes out"=w1167:i64, "Control-Client out"=w1170:refnum<class "Control-Client.lvclass">)  [unwired: 6 in]
          }
          event "StartButton": Value Change {
            n117 = event-data() -> ("NewVal"=w1175:bool)  [unwired: 1 in, 4 out]
            n118 = Not(x=w1175) -> (.not. x?=w1174:bool)
          }
          event User Event {
            n119 = event-data() -> ("command"=w1185:string, "data"=w1186:variant)  [unwired: 1 in, 4 out]
            n120 = case shown="\"UPDATE:Control\"" w1185 {
              tunnel: w1186 -> [_ w1192]
              tunnel: [w1188 w1191] -> w1182
              tunnel: w1184 -> [w1188 _]
              tunnel: w1183 -> [w1187 w1190]
              tunnel: [w1187 w1189] -> w1181
              frame "False", Default {
              }
              frame "UPDATE:Control" {
                n121 = Variant To Data(error in=w1190, type=refnum<class "Control-Client.lvclass"> refnum ("Control-Client.lvclass"), Variant=w1192) -> (data=w1191:refnum<class "Control-Client.lvclass">, error out=w1189:errorcluster)
              }
            }
            n122 = call "Set error.vi"("error in (no error)"=w1181, "Control-Client in"=w1182) -> ("error out"=w1179:errorcluster, "Control-Client out"=w1180:refnum<class "Control-Client.lvclass">)  [unwired: 8 in]
          }
        }
        "bytes received" <- w1158
      }
      n123 = while "Control Loop" {
        tunnel: w135 -> [w235]
        shift-right: [w230] -> _
        shift-left: w134 -> [w234]
        tunnel: w136 -> [w231]
        shift-right: [w226] -> _
        shift-left: 0 -> [w228]
        stop <- w233 stop-if-true
        # "Control loop"
        n124 = event shown="[51] \"Oscilloscope\": Cursor Move" {
          selector: w231 -> [_ _ _ _ _ _ _ _ _ _ _ _ _ _ _ _ _ _ _ _ _ _ _ _ _ _ _ _ _ _ _ _ _ _ _ _ _ _ _ _ _ _ _ _ _ _ _ _ _ _ _ _ _ _ _ _ _ _ _ _ _ _ _ _]
          dyn-events: _ -> [_ _ _ _ _ _ _ _ _ _ _ _ _ _ _ _ _ _ _ _ _ _ _ _ _ _ _ _ _ _ _ _ _ _ _ _ _ _ _ _ _ _ _ _ _ _ _ _ _ _ _ _ _ _ _ _ _ _ _ _ _ _ _ _]
          timeout: 10 -> [_ _ _ _ _ _ _ _ _ _ _ _ _ _ _ _ _ _ _ _ _ _ _ _ _ _ _ _ _ _ _ _ _ _ _ _ _ _ _ _ _ _ _ _ _ _ _ _ _ _ _ _ _ _ _ _ _ _ _ _ _ _ _ _]
          tunnel: w235 -> [w240 w251 w263 w279 w316 w326 w338 w365 w378 w387 w402 w415 w427 w444 w450 w469 w474 w479 w489 w501 w511 w528 w561 w574 w586 w596 w599 w605 w615 w639 w677 w689 w718 w734 w749 w762 w780 w799 w807 w819 w825 w845 w868 w883 w905 w922 w926 w930 w957 w971 w983 w992 w995 w1002 w1035 w1039 w1054 w1064 w1086 w1095 w1120 w1135 w1139 w1149]
          tunnel: [w241 w251 w258 w280 w315 w324 w336 w367 w376 w388 w400 w416 w430 w443 w447 w468 w471 w478 w488 w500 w512 w524 w559 w572 w585 w596 w599 w604 w614 w637 w678 w690 w719 w733 w747 w760 w778 w799 w806 w817 w824 w844 w866 w881 w904 w922 w925 w929 w955 w968 w980 w990 w996 w1001 w1034 w1038 w1055 w1066 w1086 w1096 w1119 w1132 w1138 w1148] -> _
          tunnel: w234 -> [w242 w252 w262 w281 w314 w325 w339 w364 w379 w390 w403 w418 w428 w445 w449 w470 w475 w480 w490 w502 w514 w526 w562 w575 w587 w597 w600 w606 w616 w640 w680 w692 w721 w735 w750 w763 w781 w800 w804 w820 w826 w846 w869 w884 w906 w923 w927 w931 w958 w970 w984 w993 w998 w1003 w1036 w1041 w1052 w1065 w1087 w1098 w1121 w1134 w1136 w1151]
          tunnel: [w239 w252 w259 w282 w313 w323 w337 w366 w377 w389 w401 w417 w429 w442 w448 w467 w473 w476 w487 w499 w513 w525 w560 w573 w588 w597 w600 w603 w613 w638 w679 w691 w720 w732 w748 w761 w779 w800 w805 w818 w823 w843 w867 w880 w903 w923 w924 w928 w956 w969 w981 w991 w997 w1004 w1033 w1040 w1053 w1067 w1087 w1097 w1118 w1133 w1137 w1147] -> w230
          tunnel: [_ _ _ w278 _ _ _ _ _ _ _ _ _ _ _ _ _ _ _ _ _ _ _ _ _ _ _ _ _ _ _ _ _ _ _ _ _ _ _ _ _ _ _ _ _ _ _ _ _ _ _ _ _ _ _ _ _ _ _ _ _ _ _ _] -> w233
          event Timeout {
            n125 = event-data() -> ()  [unwired: 1 in, 1 out]
            n126 = flat-sequence {
              tunnel: [w250] -> w239
              tunnel: w242 -> [w249]
              tunnel: [w248] -> w241
              tunnel: w240 -> [w247]
              frame #0 {
                n127 = call "Execute received commands.vi"("error in (no error)"=w247, "repump"="Repump", "Control-Client in"=w249) -> ("error out"=w244:errorcluster, "Control-Client out"=w246:refnum<class "Control-Client.lvclass">)  [unwired: 7 in]
                n128 = call "Update control status.vi"("error in (no error)"=w247, "Control-Client old"=w249, "Control-Client new"=w246) -> ("error out"=w245:errorcluster, "Control-Client en sortie"=w250:refnum<class "Control-Client.lvclass">)  [unwired: 7 in]
                n129 = Merge Errors(w245, w244) -> (w248:errorcluster)
              }
            }
          }
          event "type of probe": Value Change {
            n130 = event-data() -> ("NewVal"=w253:enum32{"SC", "OPA"})  [unwired: 1 in, 5 out]
            n131 = case shown="\"SC\", Default" w253 {
              frame "OPA" {
                n132 = global write "globalVarII.vi" "DL_n_passes"(2 ("DL_n_passes")) -> ()
                n133 = global write "globalVarII.vi" "DL_axis"(4 ("DL_axis")) -> ()
              }
              frame "SC", Default {
                n134 = global write "globalVarII.vi" "DL_n_passes"(4 ("DL_n_passes")) -> ()
                n135 = global write "globalVarII.vi" "DL_axis"(2 ("DL_axis")) -> ()
              }
            }
          }
          event "EXP": Value Change {
            n136 = event-data() -> ("OldVal"=w261:bool, "NewVal"=w260:bool)  [unwired: 1 in, 4 out]
            n137 = flat-sequence {
              tunnel: w263 -> [w273]
              tunnel: w262 -> [w272]
              tunnel: w261 -> [w271]
              tunnel: w260 -> [w270]
              tunnel: [w265] -> w259
              tunnel: [w264] -> w258
              frame #0 {
                n138 = call-dynamic "Read refs_controls_V0_VD2.vi"("error in (no error)"=w273, "EXP"=w271, "Control-Client in"=w272) -> ("error out"=w268:errorcluster, "refs_controls"=w267:refnum<vi>[], "Control-Client out"=w269:refnum<class "Control-Client.lvclass">)  [unwired: 6 in]
                n139 = for {
                  tunnel: w267 -> [w277] mode=indexing
                  n140 = property class="Ctl"(reference=w277, "Visible"=FALSE) -> ()  [unwired: 1 in, 2 out]
                }
                n141 = call-dynamic "Read refs_controls_V0_VD2.vi"("error in (no error)"=w268, "EXP"=w270, "Control-Client in"=w269) -> ("error out"=w264:errorcluster, "refs_controls"=w266:refnum<vi>[], "Control-Client out"=w265:refnum<class "Control-Client.lvclass">)  [unwired: 6 in]
                n142 = for {
                  tunnel: w266 -> [w275] mode=indexing
                  n143 = property class="Ctl"(reference=w275, "Visible"=TRUE) -> ()  [unwired: 1 in, 2 out]
                }
              }
            }
          }
          event "StartButton": Value Change {
            n144 = event-data() -> ("NewVal"=w283:bool)  [unwired: 1 in]
            n145 = case shown="False" w283 {
              selector: w283 -> [w289 _]
              tunnel: [w287 w310] -> w282
              tunnel: w281 -> [w291 w310]
              tunnel: [w285 w311] -> w280
              tunnel: w279 -> [w290 w311]
              tunnel: [w288 FALSE] -> w278
              frame False {
                n146 = flat-sequence {
                  tunnel: w291 -> [w306]
                  tunnel: w290 -> [w305]
                  tunnel: w289 -> [w304]
                  tunnel: [w295] -> w288
                  tunnel: [w294] -> w286
                  tunnel: [w293] -> w284
                  tunnel: [w309] -> w287
                  tunnel: w286 -> [w309]
                  tunnel: [w308] -> w285
                  tunnel: w284 -> [w308]
                  frame #0 {
                    n147 = control-ref of="This VI"() -> (w301:refnum<vi>)
                    n148 = call-dynamic "Stop.vi"("error in (no error)"=w305, "Control-Client in"=w306) -> ("error out"=w300:errorcluster, "Control-Client out"=w296:refnum<class "Control-Client.lvclass">)  [unwired: 8 in]
                    n149 = invoke class="VI" method="Default Vals.Reinit All"(reference=w301, error in=w300) -> (reference out=w302:refnum<vi>, error out=w303:errorcluster)  [unwired: 1 in, 1 out]
                    n150 = Close Reference(reference=w302, error in (no error)=w303) -> (error out=w297:errorcluster)
                    n151 = Not(x=w304) -> (.not. x?=w295:bool)
                    n152 = call "SendCommand.vi"("Message type"=T32 "Extra", "error in (no error)"=w297, "data"=variant, "Command"=T33 "SHUTDOWN" ("Commands"), "Control-Client in"=w296) -> ("error out"=w293:errorcluster, "Control-Client out"=w294:refnum<class "Control-Client.lvclass">)  [unwired: 5 in]
                  }
                  frame #1 {
                    n153 = Wait (ms)(milliseconds to wait=u32 50) -> ()  [unwired: 1 out]
                  }
                }
              }
              frame True {
              }
            }
          }
          event Mouse Up {
            n154 = event-data() -> ()  [unwired: 1 in, 1 out]
            n155 = flat-sequence {
              tunnel: w316 -> [w322]
              tunnel: [w318] -> w315
              tunnel: w314 -> [w321]
              tunnel: [w319] -> w313
              frame #0 {
                n156 = call "Add ExpGroup.vi"("error in (no error)"=w322, "folder of the day"="folder of the day", "Group title"="Group title", "Control-Client in"=w321) -> ("error out"=w318:errorcluster, "Control-Client out"=w319:refnum<class "Control-Client.lvclass">)  [unwired: 6 in]
              }
            }
          }
          event Mouse Down {
            n157 = event-data() -> ()  [unwired: 1 in, 1 out]
            n158 = flat-sequence {
              tunnel: w326 -> [w334]
              tunnel: w325 -> [w333]
              tunnel: [w332] -> w324
              tunnel: [w331] -> w323
              frame #0 {
                n159 = call "Del ExpGroup.vi"("error in (no error)"=w334, "Control-Client in"=w333) -> ("error out"=w327:errorcluster, "Control-Client out"=w328:refnum<class "Control-Client.lvclass">)  [unwired: 8 in]
                n160 = call "Update Client Data Representation.vi"("error in (no error)"=w327, "Control-Client in"=w328) -> ("error out"=w330:errorcluster, "Control-Client out"=w329:refnum<class "Control-Client.lvclass">)  [unwired: 8 in]
                n161 = call "Redraw graphs.vi"("error in (no error)"=w330, "Control-Client in"=w329) -> ("error out"=w332:errorcluster, "Control-Client out"=w331:refnum<class "Control-Client.lvclass">)  [unwired: 8 in]
              }
            }
          }
          event Value Change {
            n162 = event-data() -> ("NewVal"=w335:T10)  [unwired: 1 in]
            n163 = case shown="True" w335 {
              tunnel: w339 -> [w341 w363]
              tunnel: w338 -> [w340 w362]
              tunnel: [w341 w361] -> w337
              tunnel: [w340 w360] -> w336
              frame False {
              }
              frame True {
                n164 = local read "waves slider"() -> (w349:T11)
                n165 = local read "times slider"() -> (w346:T11)
                n166 = Unbundle(w346) -> (w345:dbl, w344:dbl)
                n167 = Unbundle(w349) -> (w348:dbl, w347:dbl)
                n168 = local read "# points"() -> (w359:i32)
                n169 = local read "Step, ps"() -> (w358:dbl)
                n170 = local read "OZ, ps"() -> (w357:dbl)
                n171 = Bundle "bounds"(w345, w344, w348, w347) -> (w353:cluster{dbl, dbl, dbl, dbl})  [unwired: 1 in]
                n172 = Bundle By Name(cluster=T34 {"Fix"=TRUE, "DeltaT"=0.0, "#points"=0, "Delay"=0.0, "output cluster"={"From Time"=0.0, "To Time"=0.0, "From Wave"=0.0, "To Wave"=0.0}}, "DeltaT"=w358, "#points"=w359, "Delay"=w357, "output cluster"=w353) -> (w342:T34)
                n173 = call "Add Exp.vi"("Parameters"=w342, "error in (no error)"=w362, "Exp name"="Exp name", "Commentaires exp"="Commentaires exp", "Control-Client in"=w363) -> ("error out"=w354:errorcluster, "Control-Client out"=w355:refnum<class "Control-Client.lvclass">)  [unwired: 5 in]
                n174 = call "Update Client Data Representation.vi"("error in (no error)"=w354, "Control-Client in"=w355) -> ("error out"=w352:errorcluster, "Control-Client out"=w351:refnum<class "Control-Client.lvclass">)  [unwired: 8 in]
                n175 = call "Redraw graphs.vi"("error in (no error)"=w352, "Control-Client in"=w351) -> ("error out"=w360:errorcluster, "Control-Client out"=w361:refnum<class "Control-Client.lvclass">)  [unwired: 8 in]
              }
            }
          }
          event Mouse Up {
            n176 = event-data() -> ()  [unwired: 1 in, 1 out]
            n177 = flat-sequence {
              tunnel: [w375] -> w367
              tunnel: [w374] -> w366
              tunnel: w365 -> [w373]
              tunnel: w364 -> [w372]
              frame #0 {
                n178 = call "Del Exp.vi"("error in (no error)"=w373, "Control-Client in"=w372) -> ("error out"=w370:errorcluster, "Control-Client out"=w371:refnum<class "Control-Client.lvclass">)  [unwired: 8 in]
                n179 = call "Update Client Data Representation.vi"("error in (no error)"=w370, "Control-Client in"=w371) -> ("error out"=w369:errorcluster, "Control-Client out"=w368:refnum<class "Control-Client.lvclass">)  [unwired: 8 in]
                n180 = call "Redraw graphs.vi"("error in (no error)"=w369, "Control-Client in"=w368) -> ("error out"=w375:errorcluster, "Control-Client out"=w374:refnum<class "Control-Client.lvclass">)  [unwired: 8 in]
              }
            }
          }
          event Mouse Up {
            n181 = event-data() -> ()  [unwired: 1 in, 1 out]
            n182 = flat-sequence {
              tunnel: w379 -> [w386]
              tunnel: w378 -> [w385]
              tunnel: [w384] -> w377
              tunnel: [w383] -> w376
              frame #0 {
                n183 = local read "Exp name"() -> (w382:string)
                n184 = call "Rename Exp.vi"("error in (no error)"=w385, "New exp name"=w382, "Control-Client in"=w386) -> ("error out"=w380:errorcluster, "Control-Client out"=w381:refnum<class "Control-Client.lvclass">)  [unwired: 7 in]
                n185 = call "Update Client Data Representation.vi"("error in (no error)"=w380, "Control-Client in"=w381) -> ("error out"=w383:errorcluster, "Control-Client out"=w384:refnum<class "Control-Client.lvclass">)  [unwired: 8 in]
              }
            }
          }
          event Value Change {
            n186 = event-data() -> ("NewVal"=w391:T13)  [unwired: 1 in]
            n187 = case shown="True" w391 {
              tunnel: w390 -> [w393 w398]
              tunnel: [w393 w397] -> w389
              tunnel: [w392 w394] -> w388
              tunnel: w387 -> [w392 w396]
              frame False {
              }
              frame True {
                n188 = call "Save exp.vi"("error in (no error)"=w396, "save"="Save", "Control-Client in"=w398) -> ("error out"=w394:errorcluster, "Control-Client out"=w397:refnum<class "Control-Client.lvclass">)  [unwired: 7 in]
              }
            }
          }
          event Value Change {
            n189 = event-data() -> ("NewVal"=w399:T12)  [unwired: 1 in]
            n190 = case shown="True" w399 {
              tunnel: w403 -> [w405 w414]
              tunnel: w402 -> [w404 w413]
              tunnel: [w405 w407] -> w401
              tunnel: [w404 w408] -> w400
              frame False {
              }
              frame True {
                n191 = call "Load exp.vi"("error in (no error)"=w413, "Files of Type"=string[][] [["*.dat", "DAT"], ["*.zip", "ZIP RAW"], ["*.img", "IMG"], ["*.his", "HIS"], ["*.*", "All Files"]], "Control-Client in"=w414) -> ("error out"=w410:errorcluster, "Control-Client out"=w411:refnum<class "Control-Client.lvclass">)  [unwired: 7 in]
                n192 = call "Update Client Data Representation.vi"("error in (no error)"=w410, "Control-Client in"=w411) -> ("error out"=w409:errorcluster, "Control-Client out"=w412:refnum<class "Control-Client.lvclass">)  [unwired: 8 in]
                n193 = call "Redraw graphs.vi"("error in (no error)"=w409, "Control-Client in"=w412) -> ("error out"=w408:errorcluster, "Control-Client out"=w407:refnum<class "Control-Client.lvclass">)  [unwired: 8 in]
              }
            }
          }
          event Value Change {
            n194 = event-data() -> ("NewVal"=w419:T7)  [unwired: 1 in]
            n195 = case shown="True" w419 {
              tunnel: [w421 w424] -> w417
              tunnel: w418 -> [w421 w423]
              tunnel: [w420 w425] -> w416
              tunnel: w415 -> [w420 w426]
              frame False {
              }
              frame True {
                n196 = call "CalcStability.vi"("error in (no error)"=w426, "Control-Client in"=w423) -> ("error out"=w425:errorcluster, "stability"=→"stability":T8, "Control-Client out"=w424:refnum<class "Control-Client.lvclass">)  [unwired: 7 in]
              }
            }
          }
          event "Group": Value Change {
            n197 = event-data() -> ("NewVal"=w431:u16)  [unwired: 1 in]
            n198 = flat-sequence {
              tunnel: w431 -> [w436]
              tunnel: [w432] -> w430
              tunnel: [w433] -> w429
              tunnel: w428 -> [w438]
              tunnel: w427 -> [w437]
              frame #0 {
                n199 = call "Write Group #.vi"("error in (no error)"=w437, "Group #"=w436, "Control-Client in"=w438) -> ("error out"=w440:errorcluster, "Control-Client out"=w439:refnum<class "Control-Client.lvclass">)  [unwired: 7 in]
                n200 = call "Update Client Data Representation.vi"("error in (no error)"=w440, "Control-Client in"=w439) -> ("error out"=w435:errorcluster, "Control-Client out"=w434:refnum<class "Control-Client.lvclass">)  [unwired: 8 in]
                n201 = call "Redraw graphs.vi"("error in (no error)"=w435, "Control-Client in"=w434) -> ("error out"=w432:errorcluster, "Control-Client out"=w433:refnum<class "Control-Client.lvclass">)  [unwired: 8 in]
              }
            }
          }
          event Edit Cell {
            n202 = event-data() -> ("Row"=w441:i32, "String"=w446:string)  [unwired: 1 in]
            n203 = call "Update name of exp.vi"("error in (no error)"=w444, "Exp name"=w446, "Exp #"=w441, "Control-Client in"=w445) -> ("error out"=w443:errorcluster, "Control-Client out"=w442:refnum<class "Control-Client.lvclass">)  [unwired: 6 in]
          }
          event Double Click {
            n204 = event-data() -> ("Row"=w451:i32)  [unwired: 1 in]
            n205 = stacked-sequence {
              tunnel: w451 -> [w464]
              tunnel: w450 -> [w462]
              tunnel: w449 -> [w461]
              tunnel: [w452] -> w448
              tunnel: [w453] -> w447
              frame #0 {
                n206 = call "Read Element of Exp Groups.vi"("error in (no error)"=w462, "Control-Client in"=w461) -> ("error out"=w463:errorcluster, "Experiments_group.lvclass"=w465:refnum<class "Experiments_group.lvclass">, "Control-Client out"=w459:refnum<class "Control-Client.lvclass">)  [unwired: 7 in]
                n207 = call "Set Exp sel #.vi"("error in (no error)"=w463, "Exp sel #"=w464, "Experiments_group in"=w465) -> ("error out"=w458:errorcluster, "Experiments_group out"=w460:refnum<class "Experiments_group.lvclass">)  [unwired: 7 in]
                n208 = call "Write Element of Exp Groups.vi"("error in (no error)"=w458, "Experiments_group.lvclass"=w460, "Control-Client in"=w459) -> ("error out"=w457:errorcluster, "Control-Client out"=w456:refnum<class "Control-Client.lvclass">)  [unwired: 7 in]
                n209 = call "Update Client Data Representation.vi"("error in (no error)"=w457, "Control-Client in"=w456) -> ("error out"=w454:errorcluster, "Control-Client out"=w455:refnum<class "Control-Client.lvclass">)  [unwired: 8 in]
                n210 = call "Redraw graphs.vi"("error in (no error)"=w454, "Control-Client in"=w455) -> ("error out"=w453:errorcluster, "Control-Client out"=w452:refnum<class "Control-Client.lvclass">)  [unwired: 8 in]
              }
            }
          }
          event "Commentaires exp": Value Change {
            n211 = event-data() -> ("NewVal"=w466:string)  [unwired: 1 in]
            n212 = call "Update comments exp.vi"("error in (no error)"=w469, "Commentaires"=w466, "Control-Client in"=w470) -> ("error out"=w468:errorcluster, "Control-Client out"=w467:refnum<class "Control-Client.lvclass">)  [unwired: 7 in]
          }
          event "Exp data graph": Cursor Move {
            n213 = event-data() -> ()  [unwired: 1 in, 1 out]
            n214 = call "Redraw graphs.vi"("error in (no error)"=w474, "ChangeAll"="ChangeAll", "Control-Client in"=w475) -> ("error out"=w471:errorcluster, "Control-Client out"=w473:refnum<class "Control-Client.lvclass">)  [unwired: 7 in]
          }
          event "Exp data graph": Shortcut Menu Selection (User) {
            n215 = event-data() -> ("ItemTag"=w477:string)  [unwired: 1 in]
            n216 = flat-sequence {
              tunnel: w480 -> [w486]
              tunnel: w479 -> [w485]
              tunnel: [w484] -> w478
              tunnel: [w483] -> w476
              tunnel: w477 -> [w482]
              frame #0 {
                n217 = call "Copy exp data.vi"("error in (no error)"=w485, "selected wavelengths"="selected wavelengths", "ItemTag"=w482, "Control-Client in"=w486) -> ("error out"=w484:errorcluster, "Control-Client out"=w483:refnum<class "Control-Client.lvclass">)  [unwired: 6 in]
              }
            }
          }
          event Value Change {
            n218 = event-data() -> ("NewVal"=w491:T10)  [unwired: 1 in]
            n219 = case shown="True" w491 {
              tunnel: w490 -> [w493 w498]
              tunnel: w489 -> [w492 w497]
              tunnel: [w492 w496] -> w488
              tunnel: [w493 w495] -> w487
              frame False {
              }
              frame True {
                n220 = call "Add graph.vi"("error in (no error)"=w497, "Combo Box"="Kinetics", "Control-Client in"=w498) -> ("error out"=w496:errorcluster, "Control-Client out"=w495:refnum<class "Control-Client.lvclass">)  [unwired: 7 in]
              }
            }
          }
          event Value Change {
            n221 = event-data() -> ("NewVal"=w503:T10)  [unwired: 1 in]
            n222 = case shown="True" w503 {
              tunnel: w502 -> [w505 w510]
              tunnel: w501 -> [w504 w509]
              tunnel: [w504 w508] -> w500
              tunnel: [w505 w507] -> w499
              frame False {
              }
              frame True {
                n223 = call "Add graph.vi"("error in (no error)"=w509, "Combo Box"="Spectra", "Control-Client in"=w510) -> ("error out"=w508:errorcluster, "Control-Client out"=w507:refnum<class "Control-Client.lvclass">)  [unwired: 7 in]
              }
            }
          }
          event Value Change {
            n224 = event-data() -> ("NewVal"=w515:T3)  [unwired: 1 in, 5 out]
            n225 = case shown="True" w515 {
              tunnel: w514 -> [w517 w523]
              tunnel: [w517 w522] -> w513
              tunnel: [w516 w521] -> w512
              tunnel: w511 -> [w516 w520]
              frame False {
              }
              frame True {
                n226 = local read "del kin"() -> (w518:i32)
                n227 = call "Norm graph.vi"("error in (no error)"=w520, "#kinetics"=w518, "Combo Box"="Kinetics", "Control-Client in"=w523) -> ("error out"=w521:errorcluster, "Control-Client out"=w522:refnum<class "Control-Client.lvclass">)  [unwired: 6 in]
              }
            }
          }
          event Value Change {
            n228 = event-data() -> ("CtlRef"=w529:refnum<vi>, "NewVal"=w527:variant)  [unwired: 1 in]
            n229 = flat-sequence {
              tunnel: w529 -> [w539]
              tunnel: w528 -> [w538]
              tunnel: w527 -> [w537]
              tunnel: w526 -> [w534]
              tunnel: [w533] -> w525
              tunnel: [w532] -> w524
              frame #0 {
                n230 = property class="Bool (strict)"(reference=w539, error in=w538) -> (error out=w536:errorcluster, "ClassName"=w530:string)  [unwired: 1 out]
                n231 = case shown="\"Boolean\"" w530 {
                  tunnel: [TRUE w554] -> w535
                  tunnel: [w552 w557] -> w531
                  tunnel: w537 -> [_ w556]
                  tunnel: w536 -> [w552 w555]
                  frame "Digital", Default {
                    (unwired) FALSE
                  }
                  frame "Boolean" {
                    n232 = Variant To Data(error in=w555, type=TRUE, Variant=w556) -> (data=w554:bool, error out=w557:errorcluster)
                  }
                }
                n233 = case shown="True" w535 {
                  tunnel: w534 -> [w541 w549]
                  tunnel: [w541 w548] -> w533
                  tunnel: [w540 w547] -> w532
                  tunnel: w531 -> [w540 w546]
                  frame False {
                  }
                  frame True {
                    n234 = local read "del kin"() -> (w545:i32)
                    n235 = case shown="False" "Left shift kinetics" {
                      tunnel: [0.5 -0.5] -> w542
                      frame False {
                      }
                      frame True {
                      }
                    }
                    n236 = call "Shift X kinetics.vi"("shift"=w542, "error in (no error)"=w546, "#kinetics"=w545, "Combo Box"="Kinetics", "Control-Client in"=w549) -> ("error out"=w547:errorcluster, "Control-Client out"=w548:refnum<class "Control-Client.lvclass">)  [unwired: 5 in]
                  }
                }
              }
            }
          }
          event Value Change {
            n237 = event-data() -> ("NewVal"=w563:T9)  [unwired: 1 in]
            n238 = case shown="True" w563 {
              tunnel: w562 -> [w565 w571]
              tunnel: w561 -> [w564 w570]
              tunnel: [w565 w568] -> w560
              tunnel: [w564 w567] -> w559
              frame False {
              }
              frame True {
                n239 = call "Del graph.vi"("error in (no error)"=w570, "selected graph"="del kin", "Combo Box"="Kinetics", "Control-Client in"=w571) -> ("error out"=w567:errorcluster, "Control-Client out"=w568:refnum<class "Control-Client.lvclass">)  [unwired: 6 in]
              }
            }
          }
          event Value Change {
            n240 = event-data() -> ("NewVal"=w576:T9)  [unwired: 1 in]
            n241 = case shown="True" w576 {
              tunnel: w575 -> [w578 w584]
              tunnel: w574 -> [w577 w583]
              tunnel: [w578 w581] -> w573
              tunnel: [w577 w580] -> w572
              frame False {
              }
              frame True {
                n242 = call "Del graph.vi"("error in (no error)"=w583, "selected graph"="del spec", "Combo Box"="Spectra", "Control-Client in"=w584) -> ("error out"=w580:errorcluster, "Control-Client out"=w581:refnum<class "Control-Client.lvclass">)  [unwired: 6 in]
              }
            }
          }
          event "Kinetics": Shortcut Menu Selection (User) {
            n243 = event-data() -> ("ItemTag"=w589:string)  [unwired: 1 in]
            n244 = flat-sequence {
              tunnel: w589 -> [w595]
              tunnel: [w593] -> w588
              tunnel: w587 -> [w592]
              tunnel: w586 -> [w591]
              tunnel: [w590] -> w585
              frame #0 {
                n245 = call "Copy from XY graph.vi"("error in (no error)"=w591, "ItemTag"=w595, "Type of graph"="Kinetics" ("Combo Box"), "Control-Client in"=w592) -> ("error out"=w590:errorcluster, "Control-Client out"=w593:refnum<class "Control-Client.lvclass">)  [unwired: 6 in]
              }
            }
          }
          event "Spectra": Plot Attribute Change {
            n246 = event-data() -> ("PlotIdx"=w598:i32)  [unwired: 1 in]
            n247 = property on="Spectra" class="XYGraph (strict)"("Active Plot"=w598) -> ()  [unwired: 2 in, 2 out]
          }
          event "Kinetics": Plot Attribute Change {
            n248 = event-data() -> ("PlotIdx"=w601:i32)  [unwired: 1 in]
            n249 = property on="Kinetics" class="XYGraph (strict)"("Active Plot"=w601) -> ()  [unwired: 2 in, 2 out]
          }
          event "Spectra": Shortcut Menu Selection (User) {
            n250 = event-data() -> ("ItemTag"=w602:string)  [unwired: 1 in]
            n251 = flat-sequence {
              tunnel: w606 -> [w612]
              tunnel: w605 -> [w611]
              tunnel: [w610] -> w604
              tunnel: [w609] -> w603
              tunnel: w602 -> [w608]
              frame #0 {
                n252 = call "Copy from XY graph.vi"("error in (no error)"=w611, "ItemTag"=w608, "Type of graph"=T35 "Spectra" ("Combo Box"), "Control-Client in"=w612) -> ("error out"=w610:errorcluster, "Control-Client out"=w609:refnum<class "Control-Client.lvclass">)  [unwired: 6 in]
              }
            }
          }
          event Value Change {
            n253 = event-data() -> ("NewVal"=w617:T15)  [unwired: 1 in]
            n254 = case shown="True" w617 {
              tunnel: [w619 w633] -> w613
              tunnel: w616 -> [w619 w634]
              tunnel: w615 -> [w618 w631]
              tunnel: [w618 w632] -> w614
              frame False {
              }
              frame True {
                n255 = local read "waves slider"() -> (w627:T11)
                n256 = local read "times slider"() -> (w624:T11)
                n257 = property on="Commentaires exp" class="Str"() -> ("Value"=w630:string)  [unwired: 2 in, 2 out]
                n258 = property on="Exp name" class="Str"() -> ("Value"=w629:string)  [unwired: 2 in, 2 out]
                n259 = Unbundle(w624) -> (w623:dbl, w622:dbl)
                n260 = Unbundle(w627) -> (w626:dbl, w625:dbl)
                n261 = Bundle "bounds"(w623, w622, w626, w625) -> (w621:cluster{dbl, dbl, dbl, dbl})  [unwired: 1 in]
                n262 = Bundle("Value"=w629, "Value"=w630, w621) -> (w620:T38)  [unwired: 1 in]
                n263 = call "Average experiments.vi"("error in (no error)"=w631, "sigma"="sigma", "Name+Comments+bounds"=w620, "Control-Client in"=w634) -> ("error out"=w632:errorcluster, "Control-Client out"=w633:refnum<class "Control-Client.lvclass">)  [unwired: 6 in]
              }
            }
          }
          event "side p", "polynom order": Value Change {
            n264 = event-data() -> ("CtlRef"=w636:refnum<vi>, "NewVal"=w635:variant)  [unwired: 1 in]
            n265 = flat-sequence {
              tunnel: w640 -> [w652]
              tunnel: w639 -> [w646]
              tunnel: [w644] -> w638
              tunnel: [w648] -> w637
              tunnel: w636 -> [w651]
              tunnel: w635 -> [w641]
              frame #0 {
                n266 = flat-sequence {
                  tunnel: [w653] -> w642
                  tunnel: w641 -> [w653]
                  frame #0 {
                    n267 = global write "globalVarSD.vi" "BG type"("BG type") -> ()
                    n268 = global write "globalVarSD.vi" "side points BG"("side p") -> ()
                    n269 = global write "globalVarSD.vi" "polynom order BG"("polynom order") -> ()
                  }
                }
                n270 = property class="Ctl"(reference=w651) -> ("ClassName"=w650:string)  [unwired: 1 in, 2 out]
                n271 = case shown="\"Boolean\"" w650 {
                  tunnel: [FALSE w675] -> w649
                  tunnel: w642 -> [_ w676]
                  tunnel: [TRUE w674] -> w647
                  tunnel: w646 -> [w669 w673]
                  tunnel: [w669 w672] -> w645
                  frame "Digital", Default {
                  }
                  frame "Boolean" {
                    w675 = TRUE
                    n272 = Variant To Data(error in=w673, type=w675, Variant=w676) -> (data=w674:bool, error out=w672:errorcluster)
                  }
                }
                n273 = case shown="True" w647 {
                  tunnel: w652 -> [w660 w668]
                  tunnel: w645 -> [w659 w667]
                  tunnel: w649 -> [_ w666]
                  tunnel: [w660 w665] -> w643
                  tunnel: [w659 w664] -> w648
                  frame False {
                  }
                  frame True {
                    n274 = Unbundle("BG slider") -> (w661:dbl, w662:dbl)
                    n275 = call "BG correction.vi"("Change?"=w666, "error in (no error)"=w667, "def pixel upper"=w662, "def pixel lower"=w661, "Control-Client in"=w668) -> ("error out"=w664:errorcluster, "Control-Client out"=w665:refnum<class "Control-Client.lvclass">)  [unwired: 5 in]
                  }
                }
                n276 = flat-sequence {
                  tunnel: [w658] -> w644
                  tunnel: w643 -> [w658]
                  frame #0 {
                    n277 = global read "globalVarSD.vi" "Graphs BG"() -> (→"BG":cluster{i32[], "Filtered X":dbl[]}[])
                  }
                }
              }
            }
          }
          event "correct raw BG": Value Change {
            n278 = event-data() -> ("NewVal"=w681:bool)  [unwired: 1 in, 2 out]
            n279 = case shown="True" w681 {
              tunnel: w680 -> [w683 w688]
              tunnel: [w683 w687] -> w679
              tunnel: [w682 w686] -> w678
              tunnel: w677 -> [w682 w685]
              frame False {
              }
              frame True {
                n280 = call "Raw_BG_correction.vi"("error in (no error)"=w685, "raw bg"="raw bg", "Control-Client in"=w688) -> ("error out"=w686:errorcluster, "Control-Client out"=w687:refnum<class "Control-Client.lvclass">)  [unwired: 7 in]
              }
            }
          }
          event Value Change; "Kinetics": Cursor Move {
            n281 = event-data() -> ("CtlRef"=w693:refnum<vi>)  [unwired: 1 in]
            n282 = flat-sequence {
              tunnel: w693 -> [w699]
              tunnel: w692 -> [w698]
              tunnel: [w697] -> w691
              tunnel: [w696] -> w690
              tunnel: w689 -> [w695]
              frame #0 {
                n283 = property class="Ctl"(reference=w699, error in=w695) -> (error out=w694:errorcluster, "ClassName"=w703:string)  [unwired: 1 out]
                n284 = case shown="\"XYGraph\", Default" w703 {
                  tunnel: [FALSE TRUE] -> w702
                  tunnel: [TRUE "Clean"] -> w701
                  tunnel: [w712 w715] -> w700
                  tunnel: w694 -> [w712 w715]
                  frame "XYGraph", Default {
                  }
                  frame "Boolean" {
                  }
                }
                n285 = case shown="True" w701 {
                  tunnel: w700 -> [w705 w710]
                  tunnel: w702 -> [_ w709]
                  tunnel: [w705 w706] -> w696
                  tunnel: w698 -> [w704 w711]
                  tunnel: [w704 w707] -> w697
                  frame False {
                  }
                  frame True {
                    n286 = call "CursorKinGraphMove.vi"("error in (no error)"=w710, "change"=w709, "Clean mode"="Clean mode", "Control-Client in"=w711) -> ("error out"=w706:errorcluster, "Control-Client out"=w707:refnum<class "Control-Client.lvclass">)  [unwired: 6 in]
                  }
                }
              }
            }
          }
          event Value Change {
            n287 = event-data() -> ()  [unwired: 1 in, 1 out]
            n288 = flat-sequence {
              tunnel: w721 -> [w730]
              tunnel: [w729] -> w720
              tunnel: [w728] -> w719
              tunnel: w718 -> [w727]
              frame #0 {
                n289 = local read "ChangeAll"() -> (w722:T5)
                n290 = Unbundle("waves slider") -> (w724:dbl, w723:dbl)
                n291 = call "Change FromToWave_or_Time.vi"("ChangeAll"=w722, "Combo Box"=T35 "Spectra", "error in (no error)"=w727, "To"=w723, "From"=w724, "Control-Client in"=w730) -> ("error out"=w728:errorcluster, "Control-Client out"=w729:refnum<class "Control-Client.lvclass">)  [unwired: 4 in]
              }
            }
          }
          event Value Change {
            n292 = event-data() -> ("NewVal"=w731:T11)  [unwired: 1 in]
            n293 = flat-sequence {
              tunnel: w735 -> [w744]
              tunnel: [w743] -> w732
              tunnel: [w742] -> w733
              tunnel: w734 -> [w741]
              tunnel: w731 -> [_]
              frame #0 {
                n294 = local read "ChangeAll"() -> (w736:T5)
                n295 = Unbundle("times slider") -> (w737:dbl, w738:dbl)
                n296 = call "Change FromToWave_or_Time.vi"("ChangeAll"=w736, "Combo Box"=T35 "Kinetics", "error in (no error)"=w741, "To"=w738, "From"=w737, "Control-Client in"=w744) -> ("error out"=w742:errorcluster, "Control-Client out"=w743:refnum<class "Control-Client.lvclass">)  [unwired: 4 in]
              }
            }
          }
          event "OZ, ps", "Step, ps", "# points", "Real zero, ps": Value Change {
            n297 = event-data() -> ()  [unwired: 1 in, 1 out]
            n298 = flat-sequence {
              tunnel: w750 -> [w755]
              tunnel: w749 -> [w754]
              tunnel: [w753] -> w746
              tunnel: [w752] -> w745
              tunnel: [w757] -> w747
              tunnel: [w758] -> w748
              tunnel: w746 -> [w758]
              tunnel: w745 -> [w757]
              frame #0 {
                n299 = call "Set Exp Param and Set Delays.vi"("Control-Client in"=w755, "remake"="remake", "error in (no error)"=w754) -> ("Control-Client out"=w753:refnum<class "Control-Client.lvclass">, "error out"=w752:errorcluster)  [unwired: 11 in]
              }
              frame #1 {
                n300 = property on="remake" class="Bool (strict)"("Value"=FALSE ("remake")) -> ()  [unwired: 2 in, 2 out]
              }
            }
          }
          event "# par point": Value Change {
            n301 = event-data() -> ("NewVal"=w759:i32)  [unwired: 1 in, 5 out]
            n302 = flat-sequence {
              tunnel: w763 -> [w776]
              tunnel: w762 -> [w775]
              tunnel: [w774] -> w761
              tunnel: [w773] -> w760
              tunnel: w759 -> [w772]
              frame #0 {
                n303 = call "Get_right_exp.vi"("error in (no error)"=w775, "Control-Client in"=w776) -> ("error out"=w764:errorcluster, "Right experiment"=w765:refnum<class "Experiment.lvclass">, "Control-Client out"=w770:refnum<class "Control-Client.lvclass">)  [unwired: 7 in]
                n304 = call "Write #pp.vi"("error in (no error)"=w764, "#pp"=w772, "Experiment in"=w765) -> ("error out"=w766:errorcluster, "Experiment out"=w767:refnum<class "Experiment.lvclass">)  [unwired: 7 in]
                n305 = call "Form time_delays.vi"("error in (no error)"=w766, "Control-Client"=w770, "Experiment in"=w767) -> ("error out"=w769:errorcluster, "Control-Client out"=w768:refnum<class "Control-Client.lvclass">, "Experiment out"=w771:refnum<class "Experiment.lvclass">)  [unwired: 6 in]
                n306 = call "Set_right_exp.vi"("error in (no error)"=w769, "Experiment in"=w771, "Control-Client in"=w768) -> ("error out"=w773:errorcluster, "Control-Client out"=w774:refnum<class "Control-Client.lvclass">)  [unwired: 7 in]
              }
            }
          }
          event Value Change {
            n307 = event-data() -> ("NewVal"=w777:T23)  [unwired: 1 in]
            n308 = case shown="True" w777 {
              tunnel: w781 -> [w783 w798]
              tunnel: w780 -> [w782 w797]
              tunnel: [w783 w796] -> w779
              tunnel: [w782 w795] -> w778
              frame False {
              }
              frame True {
                n309 = call "Open_abscisseSD.vi"() -> ("wavelengths"=w786:dbl[])  [unwired: 1 in]
                n310 = call "Get sel exp.vi"("error in (no error)"=w797, "Control-Client in"=w798) -> ("error out"=w794:errorcluster, "Sel experiment"=w790:refnum<class "Experiment.lvclass">, "Control-Client out"=w793:refnum<class "Control-Client.lvclass">)  [unwired: 7 in]
                n311 = call "set_timedelays_exp.vi"("error in (no error)"=w794, "timedelays"=w786, "Experiment.lvclass in"=w790) -> ("error out"=w792:errorcluster, "Experiment.lvclass out"=w791:refnum<class "Experiment.lvclass">)  [unwired: 7 in]
                n312 = Array Size(array=w786) -> (size(s)=w787:i32)
                n313 = Index Array(array=w786, index=0) -> (element=w785:dbl)
                n314 = call "Set sel exp.vi"("error in (no error)"=w792, "Experiment"=w791, "Control-Client in"=w793) -> ("error out"=w788:errorcluster, "Control-Client out"=w789:refnum<class "Control-Client.lvclass">)  [unwired: 7 in]
                n315 = call "Update time delay graph.vi"("error in (no error)"=w788, "Control-Client en entrée"=w789) -> ("error out"=w795:errorcluster, "Control-Client en sortie"=w796:refnum<class "Control-Client.lvclass">)  [unwired: 8 in]
                n316 = property on="# points" class="DigNum (strict)"("Value"=w787) -> ()  [unwired: 2 in, 2 out]
                n317 = property on="OZ, ps" class="DigNum (strict)"("Value"=w785) -> ()  [unwired: 2 in, 2 out]
              }
            }
          }
          event "LogY": Value Change {
            n318 = event-data() -> ("NewVal"=w801:bool)  [unwired: 1 in]
            n319 = flat-sequence {
              tunnel: w801 -> [w803]
              frame #0 {
                n320 = Boolean To (0,1)(Boolean=w803) -> (0, 1=w802:i16)
                n321 = property on="Kinetics" class="XYGraph (strict)"("YScale.Mapping Mode"=w802) -> ()  [unwired: 2 in, 2 out]
              }
            }
          }
          event "Unlock": Value Change {
            n322 = event-data() -> ("NewVal"=w808:bool)  [unwired: 1 in]
            n323 = flat-sequence {
              tunnel: w808 -> [w815]
              tunnel: w807 -> [w814]
              tunnel: [w812] -> w806
              tunnel: [w811] -> w805
              tunnel: w804 -> [w809]
              frame #0 {
                n324 = call "Close-open permission controls.vi"("error in (no error)"=w814, "Boolean"=w815, "Control-Client in"=w809) -> ("error out"=w813:errorcluster, "Control-Client out"=w810:refnum<class "Control-Client.lvclass">)  [unwired: 7 in]
                n325 = call "Update control status.vi"("error in (no error)"=w813, "Control-Client old"=w809, "Control-Client new"=w810) -> ("error out"=w812:errorcluster, "Control-Client en sortie"=w811:refnum<class "Control-Client.lvclass">)  [unwired: 7 in]
              }
            }
          }
          event "Server ON/OFF": Value Change {
            n326 = event-data() -> ("NewVal"=w816:bool)  [unwired: 1 in]
            n327 = call "Init connection with server.vi"("error in (no error)"=w819, "Boolean"=w816, "Control-Client in"=w820) -> ("error out"=w817:errorcluster, "Control-Client out"=w818:refnum<class "Control-Client.lvclass">)  [unwired: 7 in]
          }
          event "DL:Connect", "DET:Connect", "OSc:Connect", "DAQmx:Connect", "DAQmx:LaserShutter", "DAQmx:RelayKeyHeater", "DAQmx:FaradayCup", "DAQmx:AcceleratorShutter", "SERVER:AllConnect": Value Change {
            n328 = event-data() -> ("CtlRef"=w821:refnum<vi>, "NewVal"=w822:bool)  [unwired: 1 in]
            n329 = flat-sequence {
              tunnel: w826 -> [w839]
              tunnel: w825 -> [w838]
              tunnel: [w837] -> w824
              tunnel: [w836] -> w823
              tunnel: w822 -> [w835]
              tunnel: w821 -> [w834]
              frame #0 {
                n330 = property class="Bool (strict)"(reference=w834) -> ("Label.Text"=w832:string)  [unwired: 1 in, 2 out]
                n331 = Flatten To String(anything=w835, error in (no error)=w838) -> (data string=w827:string, error out=w828:errorcluster)  [unwired: 2 in, 1 out]
                n332 = Concatenate Strings("CLIENT:" ("chaîne"), w832) -> (w831:string)
                n333 = To Variant(anything=w827) -> (Variant=w830:variant)
                n334 = call "SendCommand.vi"("Message type"=T32 "Control", "error in (no error)"=w828, "data"=w830, "Command"=w831, "Control-Client in"=w839) -> ("error out"=w837:errorcluster, "Control-Client out"=w836:refnum<class "Control-Client.lvclass">)  [unwired: 5 in]
              }
            }
          }
          event User Event {
            n335 = event-data() -> ("DL pos"=w842:dbl, "Cell number"=w841:i32, "axis"=w840:i32)  [unwired: 1 in, 4 out]
            n336 = flat-sequence {
              tunnel: [w848] -> w844
              tunnel: w845 -> [w855]
              tunnel: w846 -> [w856]
              tunnel: [w850] -> w843
              tunnel: w842 -> [w854]
              tunnel: w841 -> [w852]
              tunnel: w840 -> [w847]
              frame #0 {
                n337 = call "Move Axis_G.vi"("error in (no error)"=w855, "Where, mm"=w854, "Axis"=w847, "Control-Client in"=w856) -> ("error out"=w849:errorcluster, "Control-Client out"=w851:refnum<class "Control-Client.lvclass">)  [unwired: 6 in]
                n338 = case shown="True" "Define Names" {
                  tunnel: w852 -> [_ w860]
                  tunnel: w851 -> [w858 w865]
                  tunnel: [w858 w864] -> w850
                  tunnel: w849 -> [w857 w863]
                  tunnel: [w857 w862] -> w848
                  tunnel: w847 -> [_ w859]
                  frame False {
                  }
                  frame True {
                    n339 = call-dynamic "Read Element of Names of Cells.vi"("error in (no error)"=w863, "axis"=w859, "index"=w860, "Control-Client in"=w865) -> ("error out"=w862:errorcluster, "String"=w861:string, "Control-Client out"=w864:refnum<class "Control-Client.lvclass">)  [unwired: 5 in]
                    n340 = property on="Exp name" class="Str"("Value"=w861) -> ()  [unwired: 2 in, 2 out]
                  }
                }
              }
            }
          }
          event "DAQmx:MoveCrystal": Value Change {
            n341 = event-data() -> ()  [unwired: 1 in, 6 out]
            n342 = flat-sequence {
              tunnel: [w878] -> w866
              tunnel: w868 -> [w873]
              tunnel: w869 -> [w875]
              tunnel: [w874] -> w867
              frame #0 {
                n343 = Flatten To String(anything="Time, ms", error in (no error)=w873) -> (data string=w871:string, error out=w872:errorcluster)  [unwired: 2 in, 1 out]
                n344 = To Variant(anything=w871) -> (Variant=w877:variant)
                n345 = call "SendCommand.vi"("Message type"=T32 "Control", "error in (no error)"=w872, "data"=w877, "Command"=T33 "CLIENT:DAQmx:MoveCrystal" ("Commands"), "Control-Client in"=w875) -> ("error out"=w878:errorcluster, "Control-Client out"=w874:refnum<class "Control-Client.lvclass">)  [unwired: 5 in]
              }
            }
          }
          event "RT": Value Change {
            n346 = event-data() -> ("NewVal"=w882:bool)  [unwired: 1 in, 5 out]
            n347 = flat-sequence {
              tunnel: w884 -> [w891]
              tunnel: w883 -> [w889]
              tunnel: w882 -> [w887]
              tunnel: [w885] -> w881
              tunnel: [w886] -> w880
              frame #0 {
                n348 = call "Write RT.vi"("error in (no error)"=w889, "RT"=w887, "Control-Client in"=w891) -> ("error out"=w890:errorcluster, "Control-Client out"=w888:refnum<class "Control-Client.lvclass">)  [unwired: 7 in]
                n349 = case shown="True" w887 {
                  tunnel: w888 -> [w893 w895]
                  tunnel: w890 -> [w892 w898]
                  tunnel: [w892 w897] -> w885
                  tunnel: [w893 w896] -> w886
                  frame False {
                  }
                  frame True {
                    n350 = call "Measure_G.vi"("All"=TRUE, "error in (no error)"=w898, "repump_correction"=FALSE ("All"), "# scans"="# par point", "Control-Client in"=w895) -> ("error out"=w897:errorcluster, "Control-Client out"=w896:refnum<class "Control-Client.lvclass">)  [unwired: 5 in]
                  }
                }
              }
            }
          }
          event "Start measurement": Value Change {
            n351 = event-data() -> ("NewVal"=w907:bool)  [unwired: 1 in]
            n352 = flat-sequence {
              tunnel: w907 -> [w918]
              tunnel: w906 -> [w911]
              tunnel: w905 -> [w912]
              tunnel: [w908] -> w902
              tunnel: [w909] -> w901
              tunnel: [w920] -> w903
              tunnel: [w921] -> w904
              tunnel: w902 -> [w921]
              tunnel: w901 -> [w920]
              frame #0 {
                n353 = invoke on="RT" class="Bool (strict)" method="Reinit To Default"() -> ()  [unwired: 3 in, 3 out]
                n354 = property on="Repump" class="Bool (strict)"() -> ("Value"=w910:bool)  [unwired: 2 in, 2 out]
                n355 = call "repump_state_change.vi"("error in (no error)"=w912, "repump_state"=w910, "Control-Client in"=w911) -> ("error out"=w913:errorcluster, "Control-Client out"=w914:refnum<class "Control-Client.lvclass">)  [unwired: 7 in]
                n356 = call "Write RT.vi"("error in (no error)"=w913, "RT"=FALSE, "Control-Client in"=w914) -> ("error out"=w916:errorcluster, "Control-Client out"=w917:refnum<class "Control-Client.lvclass">)  [unwired: 7 in]
                n357 = call "Write Start Meas.vi"("error in (no error)"=w916, "Start Meas"=w918, "Control-Client in"=w917) -> ("error out"=w908:errorcluster, "Control-Client out"=w909:refnum<class "Control-Client.lvclass">)  [unwired: 7 in]
              }
              frame #1 {
                n358 = Request Deallocation(TRUE ("flag")) -> ()
              }
            }
          }
          event User Event {
            n359 = event-data() -> ()  [unwired: 1 in, 5 out]
          }
          event Value Change {
            n360 = event-data() -> ()  [unwired: 1 in, 6 out]
            n361 = call "SaveSC.vi"("entrée d'erreur (pas d'erreur)"=w926, "Control-Client en entrée"=w927) -> ("sortie d'erreur"=w925:errorcluster, "Control-Client en sortie"=w924:refnum<class "Control-Client.lvclass">)  [unwired: 8 in]
          }
          event "ODmax", "ODmin", "Aq contol", "Wavelength fix", "#cycles_measurement": Value Change {
            n362 = event-data() -> ()  [unwired: 1 in, 6 out]
            n363 = flat-sequence {
              tunnel: w931 -> [w945]
              tunnel: w930 -> [w944]
              tunnel: [w935] -> w929
              tunnel: [w937] -> w928
              frame #0 {
                n364 = call "Read X-scale.vi"("error in (no error)"=w944, "Control-Client in"=w945) -> ("error out"=w936:errorcluster, "X-scale"=w943:dbl[], "Control-Client out"=w934:refnum<class "Control-Client.lvclass">)  [unwired: 7 in]
                n365 = flat-sequence {
                  tunnel: "Wavelength fix" -> [w952]
                  tunnel: w943 -> [w951]
                  tunnel: [w950] -> w939
                  frame #0 {
                    n366 = call "verify-selected-wavesSD.vi"("in wave"=w952, "wavelengths"=w951) -> ("closet wave"=w953:dbl, "closest index"=w950:i32)  [unwired: 1 in, 2 out]
                    n367 = global write "globalVarSD.vi" "wavelength fix index"(w950) -> ()
                    n368 = local write "Wavelength fix"(w953) -> ()
                  }
                }
                n369 = Bundle By Name(cluster=T36 {"ODmin"=0.0, "ODmax"=0.0, "Aq contol"=enum."fixed", "Wavelength_fix_index"=0, "repump_limits"={"repump_min"=0.0, "repump_max"=0.0, "repump_value"=0.0}, "repump_correction"=FALSE, "#cycles max"=5} ("cluster d'entrée"), "ODmin"="ODmin", "ODmax"="ODmax", "Aq contol"="Aq contol", "Wavelength_fix_index"=w939, "#cycles max"="#cycles_measurement") -> (w933:T36)
                n370 = case shown="\"automatic\"" "Aq contol" {
                  tunnel: [FALSE TRUE FALSE] -> _
                  frame "fixed", Default {
                  }
                  frame "automatic" {
                  }
                  frame "fixed-auto" {
                  }
                }
                n371 = call "Write Parameters of measurement.vi"("error in (no error)"=w936, "Paramerters of measurement d'entrée"=w933, "Control-Client en entrée"=w934) -> ("error out"=w935:errorcluster, "Control-Client en sortie"=w937:refnum<class "Control-Client.lvclass">)  [unwired: 7 in]
              }
            }
          }
          event Value Change {
            n372 = event-data() -> ("NewVal"=w954:T6)  [unwired: 1 in]
            n373 = case shown="True" w954 {
              tunnel: w958 -> [w960 w966]
              tunnel: w957 -> [w959 w965]
              tunnel: [w960 w963] -> w956
              tunnel: [w959 w964] -> w955
              frame False {
              }
              frame True {
                n374 = local read "ChangeAll"() -> (w962:T5)
                n375 = call "NaNCorrect.vi"("error in (no error)"=w965, "Value"="Value", "CorrectAll"=w962, "Control-Client in"=w966) -> ("error out"=w964:errorcluster, "Control-Client out"=w963:refnum<class "Control-Client.lvclass">)  [unwired: 6 in]
              }
            }
          }
          event Value Change {
            n376 = event-data() -> ("NewVal"=w967:T21)  [unwired: 1 in]
            n377 = flat-sequence {
              tunnel: w971 -> [w979]
              tunnel: w970 -> [w978]
              tunnel: [w975] -> w969
              tunnel: [w974] -> w968
              tunnel: w967 -> [w973]
              frame #0 {
                n378 = call "OscilloscopeRead.vi"("error in (no error)"=w979, "channelsOsc"="channelsOsc", "ON/OFF"=w973, "Control-Client in"=w978) -> ("error out"=w977:errorcluster, "Control-Client out"=w976:refnum<class "Control-Client.lvclass">)  [unwired: 6 in]
                n379 = call-dynamic "Write OscRead.vi"("error in (no error)"=w977, "OscRead"=w973, "Control-Client in"=w976) -> ("error out"=w974:errorcluster, "Control-Client out"=w975:refnum<class "Control-Client.lvclass">)  [unwired: 7 in]
              }
            }
          }
          event Value Change {
            n380 = event-data() -> ("NewVal"=w982:T19)  [unwired: 1 in]
            n381 = flat-sequence {
              tunnel: w984 -> [w989]
              tunnel: w983 -> [w988]
              tunnel: w982 -> [w987]
              tunnel: [w986] -> w981
              tunnel: [w985] -> w980
              frame #0 {
                n382 = call "StopCursorOscilloscopeMoving.vi"("error in (no error)"=w988, "Boolean"=w987, "Control-Client in"=w989) -> ("error out"=w985:errorcluster, "Control-Client out"=w986:refnum<class "Control-Client.lvclass">)  [unwired: 7 in]
              }
            }
          }
          event "Oscilloscope": Cursor Move {
            n383 = event-data() -> ()  [unwired: 1 in, 7 out]
            n384 = call "Set_WCM_limits.vi"("error in (no error)"=w992, "Control-Client in"=w993) -> ("error out"=w990:errorcluster, "Control-Client out"=w991:refnum<class "Control-Client.lvclass">)  [unwired: 8 in]
          }
          event "Repump": Value Change {
            n385 = event-data() -> ("NewVal"=w994:bool)  [unwired: 1 in]
            n386 = call "repump_state_change.vi"("error in (no error)"=w995, "repump_state"=w994, "Control-Client in"=w998) -> ("error out"=w996:errorcluster, "Control-Client out"=w997:refnum<class "Control-Client.lvclass">)  [unwired: 7 in]
          }
          event "Scale_up": Value Change {
            n387 = event-data() -> ("CtlRef"=w1000:refnum<vi>, "NewVal"=w999:variant)  [unwired: 1 in]
            n388 = flat-sequence {
              tunnel: [w1016] -> w1004
              tunnel: w1003 -> [w1015]
              tunnel: w1002 -> [w1014]
              tunnel: [w1013] -> w1001
              tunnel: w1000 -> [w1012]
              tunnel: w999 -> [w1011]
              frame #0 {
                n389 = property class="Ctl"(reference=w1012, error in=w1014) -> (error out=w1005:errorcluster, "ClassName"=w1010:string)  [unwired: 1 out]
                n390 = case shown="\"Boolean\"" w1010 {
                  tunnel: [FALSE w1032] -> w1007
                  tunnel: [TRUE w1028] -> w1006
                  tunnel: [w1025 w1031] -> w1008
                  tunnel: w1011 -> [_ w1030]
                  tunnel: w1005 -> [w1025 w1029]
                  frame "Digital", Default {
                  }
                  frame "Boolean" {
                    w1032 = TRUE
                    n391 = Variant To Data(error in=w1029, type=w1032, Variant=w1030) -> (data=w1028:bool, error out=w1031:errorcluster)
                  }
                }
                n392 = case shown="True" w1006 {
                  tunnel: w1015 -> [w1018 w1024]
                  tunnel: w1008 -> [w1017 w1023]
                  tunnel: [w1017 w1022] -> w1013
                  tunnel: [w1018 w1021] -> w1016
                  tunnel: "Scale_up" -> [_ w1020]
                  tunnel: w1007 -> [_ w1019]
                  frame False {
                  }
                  frame True {
                    n393 = call "ScaleUp correction.vi"("error in (no error)"=w1023, "Change?"=w1019, "ScaleUp"=w1020, "Control-Client in"=w1024) -> ("error out"=w1022:errorcluster, "Control-Client out"=w1021:refnum<class "Control-Client.lvclass">)  [unwired: 6 in]
                  }
                }
              }
            }
          }
          event "Define Names": Value Change {
            n394 = event-data() -> ()  [unwired: 1 in, 6 out]
            n395 = call "Define Cells names.vi"("error in (no error)"=w1035, "Control-Client in"=w1036) -> ("error out"=w1034:errorcluster, "Control-Client out"=w1033:refnum<class "Control-Client.lvclass">)  [unwired: 8 in]
          }
          event Value Change {
            n396 = event-data() -> ("NewVal"=w1037:T18)  [unwired: 1 in, 5 out]
            n397 = flat-sequence {
              tunnel: w1041 -> [w1049]
              tunnel: [w1048] -> w1040
              tunnel: w1039 -> [w1047]
              tunnel: [w1044] -> w1038
              tunnel: w1037 -> [w1042]
              frame #0 {
                n398 = call "Get VI ref.vi"("error in (no error)"=w1047, "name"="Visualize", "Control-Client in"=w1049) -> ("error out"=w1045:errorcluster, "VI ref"=w1046:refnum<vi>, "Control-Client out"=w1048:refnum<class "Control-Client.lvclass">)  [unwired: 6 in]
                n399 = invoke class="VI" method="FP.Open"(reference=w1046, error in=w1045, "Activate"=w1042, "State"=T37."Standard") -> (error out=w1044:errorcluster)  [unwired: 1 in, 4 out]
              }
            }
          }
          event "VD2_calc_abs": Value Change {
            n400 = event-data() -> ("NewVal"=w1051:bool)  [unwired: 1 in, 5 out]
            n401 = case shown="True" w1051 {
              tunnel: [w1057 w1061] -> w1055
              tunnel: w1054 -> [w1057 w1062]
              tunnel: [w1056 w1059] -> w1053
              tunnel: w1052 -> [w1056 w1060]
              frame False {
              }
              frame True {
                n402 = property on="Exp name" class="Str"() -> ("Value"=w1058:string)  [unwired: 2 in, 2 out]
                n403 = call "VD2_TRABS_Calc.vi"("error in (no error)"=w1062, "Exp name"=w1058, "Control-Client in"=w1060) -> ("error out"=w1061:errorcluster, "Control-Client out"=w1059:refnum<class "Control-Client.lvclass">)  [unwired: 7 in]
              }
            }
          }
          event "Merge": Value Change {
            n404 = event-data() -> ("NewVal"=w1063:bool)  [unwired: 1 in, 5 out]
            n405 = case shown="True" w1063 {
              tunnel: [w1069 w1082] -> w1067
              tunnel: w1065 -> [w1069 w1083]
              tunnel: w1064 -> [w1068 w1080]
              tunnel: [w1068 w1081] -> w1066
              frame False {
              }
              frame True {
                n406 = local read "waves slider"() -> (w1077:T11)
                n407 = local read "times slider"() -> (w1074:T11)
                n408 = property on="Commentaires exp" class="Str"() -> ("Value"=w1079:string)  [unwired: 2 in, 2 out]
                n409 = property on="Exp name" class="Str"() -> ("Value"=w1078:string)  [unwired: 2 in, 2 out]
                n410 = Unbundle(w1074) -> (w1073:dbl, w1072:dbl)
                n411 = Unbundle(w1077) -> (w1076:dbl, w1075:dbl)
                n412 = Bundle "bounds"(w1073, w1072, w1076, w1075) -> (w1071:cluster{dbl, dbl, dbl, dbl})  [unwired: 1 in]
                n413 = Bundle("Value"=w1078, "Value"=w1079, w1071) -> (w1070:T38)  [unwired: 1 in]
                n414 = call "Merge experiments.vi"("error in (no error)"=w1080, "Name+Comments+bounds"=w1070, "Control-Client in"=w1083) -> ("error out"=w1081:errorcluster, "Control-Client out"=w1082:refnum<class "Control-Client.lvclass">)  [unwired: 7 in]
              }
            }
          }
          event "left exp", "right exp": Value Change {
            n415 = event-data() -> ("CtlRef"=w1085:refnum<vi>, "OldVal"=w1084:bool)  [unwired: 1 in, 4 out]
            n416 = flat-sequence {
              tunnel: w1085 -> [w1092]
              tunnel: w1084 -> [w1088]
              frame #0 {
                n417 = property class="Bool (strict)"(reference=w1092) -> ("Label.Text"=w1091:string)  [unwired: 1 in, 2 out]
                n418 = Equal?(x=w1091, y="left exp") -> (x = y?=w1089:bool)
                n419 = case shown="True" w1089 {
                  tunnel: w1088 -> [w1093 w1094]
                  frame False {
                    n420 = property on="left exp" class="Bool (strict)"("Value"=w1093) -> ()  [unwired: 2 in, 2 out]
                  }
                  frame True {
                    n421 = property on="right exp" class="Bool (strict)"("Value"=w1094) -> ()  [unwired: 2 in, 2 out]
                  }
                }
              }
            }
          }
          event "Up", "Left", "Right": Value Change {
            n422 = event-data() -> ("CtlRef"=w1100:refnum<vi>, "NewVal"=w1099:bool)  [unwired: 1 in, 4 out]
            n423 = case shown="True" w1099 {
              tunnel: w1100 -> [_ w1117]
              tunnel: w1098 -> [w1101 w1109]
              tunnel: [w1101 w1108] -> w1097
              tunnel: [w1102 w1107] -> w1096
              tunnel: w1095 -> [w1102 w1106]
              frame False {
              }
              frame True {
                n424 = property class="Bool (strict)"(reference=w1117) -> ("Label.Text"=w1113:string)  [unwired: 1 in, 2 out]
                n425 = Equal?(x=w1113, y="Up") -> (x = y?=w1111:bool)
                n426 = Equal?(x=w1113, y="Left") -> (x = y?=w1103:bool)
                n427 = Equal?(x=w1113, y="Down") -> (x = y?=w1112:bool)
                n428 = Or(x=w1111, y=w1112) -> (x .or. y?=w1110:bool)
                n429 = call "Move merged.vi"("left"=w1103, "left exp"="left exp", "error in (no error)"=w1106, "vertical"=w1110, "pixel move"="Numeric", "Control-Client in"=w1109) -> ("error out"=w1107:errorcluster, "Control-Client out"=w1108:refnum<class "Control-Client.lvclass">)  [unwired: 4 in]
              }
            }
          }
          event "scale": Value Change {
            n430 = event-data() -> ("NewVal"=w1122:dbl)  [unwired: 1 in, 5 out]
            n431 = flat-sequence {
              tunnel: w1122 -> [w1131]
              tunnel: w1121 -> [w1130]
              tunnel: w1120 -> [w1129]
              tunnel: [w1128] -> w1119
              tunnel: [w1127] -> w1118
              frame #0 {
                n432 = property on="right exp" class="Bool (strict)"() -> ("Value"=w1125:bool)  [unwired: 2 in, 2 out]
                n433 = property on="left exp" class="Bool (strict)"() -> ("Value"=w1126:bool)  [unwired: 2 in, 2 out]
                n434 = Select(t=w1126, s=TRUE, f=w1125) -> (s? t:f=w1123:bool)
                n435 = call "ScaleUp merged.vi"("error in (no error)"=w1129, "left"=w1123, "scale"=w1131, "Control-Client in"=w1130) -> ("error out"=w1128:errorcluster, "Control-Client out"=w1127:refnum<class "Control-Client.lvclass">)  [unwired: 6 in]
              }
            }
          }
          event "Fix": Value Change {
            n436 = event-data() -> ()  [unwired: 1 in, 6 out]
            n437 = call "Fix merge.vi"("error in (no error)"=w1135, "Control-Client in"=w1134) -> ("error out"=w1132:errorcluster, "Control-Client out"=w1133:refnum<class "Control-Client.lvclass">)  [unwired: 8 in]
          }
          event "Cut": Value Change {
            n438 = event-data() -> ("NewVal"=w1140:bool)  [unwired: 1 in, 5 out]
            n439 = case shown="True" w1140 {
              tunnel: w1139 -> [w1141 w1146]
              tunnel: [w1141 w1145] -> w1138
              tunnel: [w1142 w1144] -> w1137
              tunnel: w1136 -> [w1142 w1143]
              frame False {
              }
              frame True {
                n440 = call "Cut merged.vi"("error in (no error)"=w1146, "Control-Client in"=w1143) -> ("error out"=w1145:errorcluster, "Control-Client out"=w1144:refnum<class "Control-Client.lvclass">)  [unwired: 8 in]
              }
            }
          }
          event "aver": Value Change {
            n441 = event-data() -> ("NewVal"=w1150:bool)  [unwired: 1 in, 5 out]
            n442 = case shown="True" w1150 {
              tunnel: w1149 -> [w1152 w1157]
              tunnel: [w1152 w1156] -> w1148
              tunnel: [w1153 w1155] -> w1147
              tunnel: w1151 -> [w1153 w1154]
              frame False {
              }
              frame True {
                n443 = call "Aver merged.vi"("error in (no error)"=w1157, "Control-Client in"=w1154) -> ("error out"=w1156:errorcluster, "Control-Client out"=w1155:refnum<class "Control-Client.lvclass">)  [unwired: 8 in]
              }
            }
          }
        }
        n444 = Increment(x=w228) -> (x+1=w225:i32)
        n445 = Greater?(x=w225, y=120000) -> (0:w227:bool)
        n446 = case shown="True" w227 {
          selector: w227 -> [_ w237]
          tunnel: [w236 0] -> w226
          tunnel: w225 -> [w236 _]
          frame False {
            (unwired) FALSE
          }
          frame True {
            n447 = Request Deallocation(w237) -> ()
          }
        }
      }
      n448 = while {
        shift-right: [w197] -> _
        shift-left: w134 -> [w200]
        tunnel: w137 -> [w196]
        tunnel: w135 -> [w199]
        tunnel: [w198] -> _
        stop <- w201 stop-if-true
        # "Send loop"
        n449 = event shown="[0] Timeout" {
          selector: w196 -> [_ _ _]
          dyn-events: _ -> [_ _ _]
          timeout: 2 -> [_ _ _]
          tunnel: [_ w206 _] -> w201
          tunnel: w200 -> [w203 w209 w215]
          tunnel: w199 -> [w205 w208 w214]
          tunnel: [w204 w208 w211] -> w198
          tunnel: [w202 w209 w212] -> w197
          event Timeout {
            n450 = event-data() -> ()  [unwired: 1 in, 3 out]
            n451 = call "Send client commands.vi"("error in (no error)"=w205, "Control-Client in"=w203) -> ("error out"=w204:errorcluster, "Control-Client out"=w202:refnum<class "Control-Client.lvclass">)  [unwired: 8 in]
          }
          event "StartButton": Value Change {
            n452 = event-data() -> ("NewVal"=w207:bool)  [unwired: 1 in, 4 out]
            n453 = Not(x=w207) -> (.not. x?=w206:bool)
          }
          event User Event {
            n454 = event-data() -> ("command"=w217:string, "data"=w216:variant)  [unwired: 1 in, 4 out]
            n455 = case shown="\"UPDATE:Control\"" w217 {
              tunnel: w216 -> [_ w223]
              tunnel: [w219 w222] -> w213
              tunnel: w215 -> [w219 _]
              tunnel: w214 -> [w218 w221]
              tunnel: [w218 w220] -> w210
              frame "False", Default {
              }
              frame "UPDATE:Control" {
                n456 = Variant To Data(error in=w221, type=refnum<class "Control-Client.lvclass"> refnum ("Control-Client.lvclass"), Variant=w223) -> (data=w222:refnum<class "Control-Client.lvclass">, error out=w220:errorcluster)
              }
            }
            n457 = call "Set error.vi"("error in (no error)"=w210, "Control-Client in"=w213) -> ("error out"=w211:errorcluster, "Control-Client out"=w212:refnum<class "Control-Client.lvclass">)  [unwired: 8 in]
          }
        }
      }
      n458 = flat-sequence {
        tunnel: w135 -> [w146]
        tunnel: w134 -> [w144]
        frame #0 {
          n459 = call <vilib>:"zmq_ctx_create.vi"("error in"=w146) -> ("error out"=w155:errorcluster, "context out"=w156:refnum<class "zmq_context.lvclass">)  [unwired: 3 in]
          n460 = call <vilib>:"zmq_socket.vi"("error in"=w155, "socket type"=socket_type."ZMQ_SUB", "context in"=w156) -> ("error out"=w154:errorcluster, "socket out"=w151:refnum<class "zmq_socket.lvclass">, "context out"=w152:refnum<class "zmq_context.lvclass">)  [unwired: 2 in]
          n461 = call <vilib>:"zmq_connect.vi"("error in"=w154, "endpoint"="tcp://129.175.100.123:5556", "socket in"=w151) -> ("error out"=w140:errorcluster, "socket out"=w143:refnum<class "zmq_socket.lvclass">)  [unwired: 1 in]
          n462 = call <vilib>:"zmq_setsocketopt.vi"("error in"=w140, "value"="", "option"=socket_options."ZMQ_SUBSCRIBE", "socket in"=w143) -> ("error out"=w141:errorcluster, "socket out"=w142:refnum<class "zmq_socket.lvclass">)  [unwired: 2 in]
          n463 = while {
            tunnel: w142 -> [w162]
            tunnel: w141 -> [w161]
            tunnel: [w158] -> w148
            tunnel: [w160] -> w147
            stop <- w159 stop-if-true
            n464 = event shown="[0] Timeout" {
              selector: _ -> [_ _]
              dyn-events: _ -> [_ _]
              timeout: 40 -> [_ _]
              tunnel: w162 -> [w167 w192]
              tunnel: w161 -> [w166 w191]
              tunnel: [w165 w192] -> w160
              tunnel: [_ w193] -> w159
              tunnel: [w164 w191] -> w158
              event Timeout {
                n465 = event-data() -> ()  [unwired: 1 in, 3 out]
                n466 = case shown="False" "image" {
                  tunnel: w167 -> [w168 w176]
                  tunnel: w166 -> [w169 w177]
                  tunnel: [w168 w181] -> w165
                  tunnel: [w169 w180] -> w164
                  frame False {
                  }
                  frame True {
                    n467 = disable-structure shown="Enabled" {
                      disable-tunnel: w177 -> [w188 w189]
                      disable-tunnel: w176 -> [w186 w190]
                      disable-tunnel: [w185 w190] -> w175
                      disable-tunnel: [w184 w189] -> w174
                      frame Disabled {
                        n468 = call <vilib>:"zmq_send.vi"("error in"=w188, "data"="giveImage" ("In"), "socket in"=w186) -> ("error out"=w184:errorcluster, "socket out"=w185:refnum<class "zmq_socket.lvclass">)  [unwired: 4 in]
                      }
                      frame Enabled {
                      }
                    }
                    n469 = call <vilib>:"zmq_recv.vi"("error in"=w174, "socket in"=w175) -> ("error out"=w178:errorcluster, "data"=w173:string, "socket out"=w181:refnum<class "zmq_socket.lvclass">)  [unwired: 3 in, 2 out]
                    n470 = Unflatten From JSON(JSON string=w173, type and defaults=dbl[][] [] ("array"), error in (no error)=w178) -> (value=w171:dbl[][], error out=w180:errorcluster)  [unwired: 4 in]
                    n471 = Transpose 2D Array(2D array=w171) -> (transposed array=w172:dbl[][])
                    n472 = for {
                      tunnel: w172 -> [w183] mode=indexing
                      tunnel: [w182] -> w170 mode=indexing
                      n473 = Reverse 1D Array(array=w183) -> (reversed array=w182:dbl[])
                    }
                    "Camera" <- w170
                  }
                }
              }
              event "StartButton": Value Change {
                n474 = event-data() -> ("NewVal"=w194:bool)  [unwired: 1 in, 5 out]
                n475 = Not(x=w194) -> (.not. x?=w193:bool)
              }
            }
          }
          n476 = call <vilib>:"zmq_close.vi"("error in"=w148, "socket"=w147) -> ("error out"=w153:errorcluster)  [unwired: 3 in]
          n477 = call <vilib>:"zmq_ctx_destroy.vi"("error in"=w153, "context in"=w152) -> ("error out"=w145:errorcluster)  [unwired: 3 in]
          n478 = call "Set error.vi"("error in (no error)"=w145, "Control-Client in"=w144) -> ()  [unwired: 8 in, 2 out]
        }
      }
    }
  }
